vi "main.vi"() -> ()   [LabVIEW 2019]
uses:
  <vilib>/Utility/miscctls.llb/LVPointTypeDef.ctl
  GitHub/ui-tools/Engine/Move Speed.ctl
  <vilib>/numeric/Random Number (Range) U64.vi
  <vilib>/numeric/sub_Random U32.vi
  <vilib>/Utility/file.llb/Read Delimited Spreadsheet (string).vi
  <vilib>/Utility/file.llb/Write Delimited Spreadsheet (string).vi
  <vilib>/Utility/file.llb/Write Delimited Spreadsheet (I64).vi
  <vilib>/Utility/file.llb/Read Delimited Spreadsheet (I64).vi
panel:
  out "倒计时":i32(slide) scale=-1.0..2181.0
  out "x-y":i32
  in  "数组":u64[](array[numeric])
  in  "Toolbar 5":T1
  in  "WindowsMediaPlayer":refnum<k7>(container)
  in  "错误输入（无错误）":errorcluster
  in  "AniGIF":refnum<k7>(container)
  in  "键盘启用":bool
  out "游戏界面_时间到":bool
  in  "亮灯次数":i32=1
  in  "是否开始计时？":bool
  out "难度":string="困难"
  out "闪烁间隔":i32=727
  out "超时时间":i32=500
  in  "选项卡控件":T2(tab)
  in  "密码:":string
  in  "账号:":string
  in  "登录界面_修改密码":bool
  in  "登陆界面_注册":bool
  in  "登录界面_登录":bool
  in  "登录界面_退出":bool
  in  "主界面_返回":bool
  in  "主界面_进入游戏":bool
  in  "用户注册_注册":bool
  in  "用户注册_返回":bool
  in  "注册簇":T3
  in  "修改密码_返回":bool
  in  "修改密码_修改":bool
  in  "修改密码簇 2":T4
  in  "TOP10_返回":bool
  out "玩家                      积分          简单":string[][](array[string])
  out "玩家                      积分          中等":string[][](array[string])
  out "玩家                      积分          困难":string[][](array[string])
  in  "TOP10_退出":bool
  in  "游戏规则_返回":bool
  out "分数":i32
  out "游戏界面_下":T5
  out "游戏界面_右":T6
  out "游戏界面_左":T7
  out "游戏界面_上":T8
  out "难度：分数":string
  in  "游戏界面_结束":bool
  out "玩家":string
  # "游戏开始时，第一次亮一\n个灯，然后我们需要点击一次已 \n，第二次会亮两个灯，包括第一\n次的灯，第三次亮三个，每次增\n加一个灯，你都需要按顺序点击\n，或者使用键盘的↑↓←→操作"
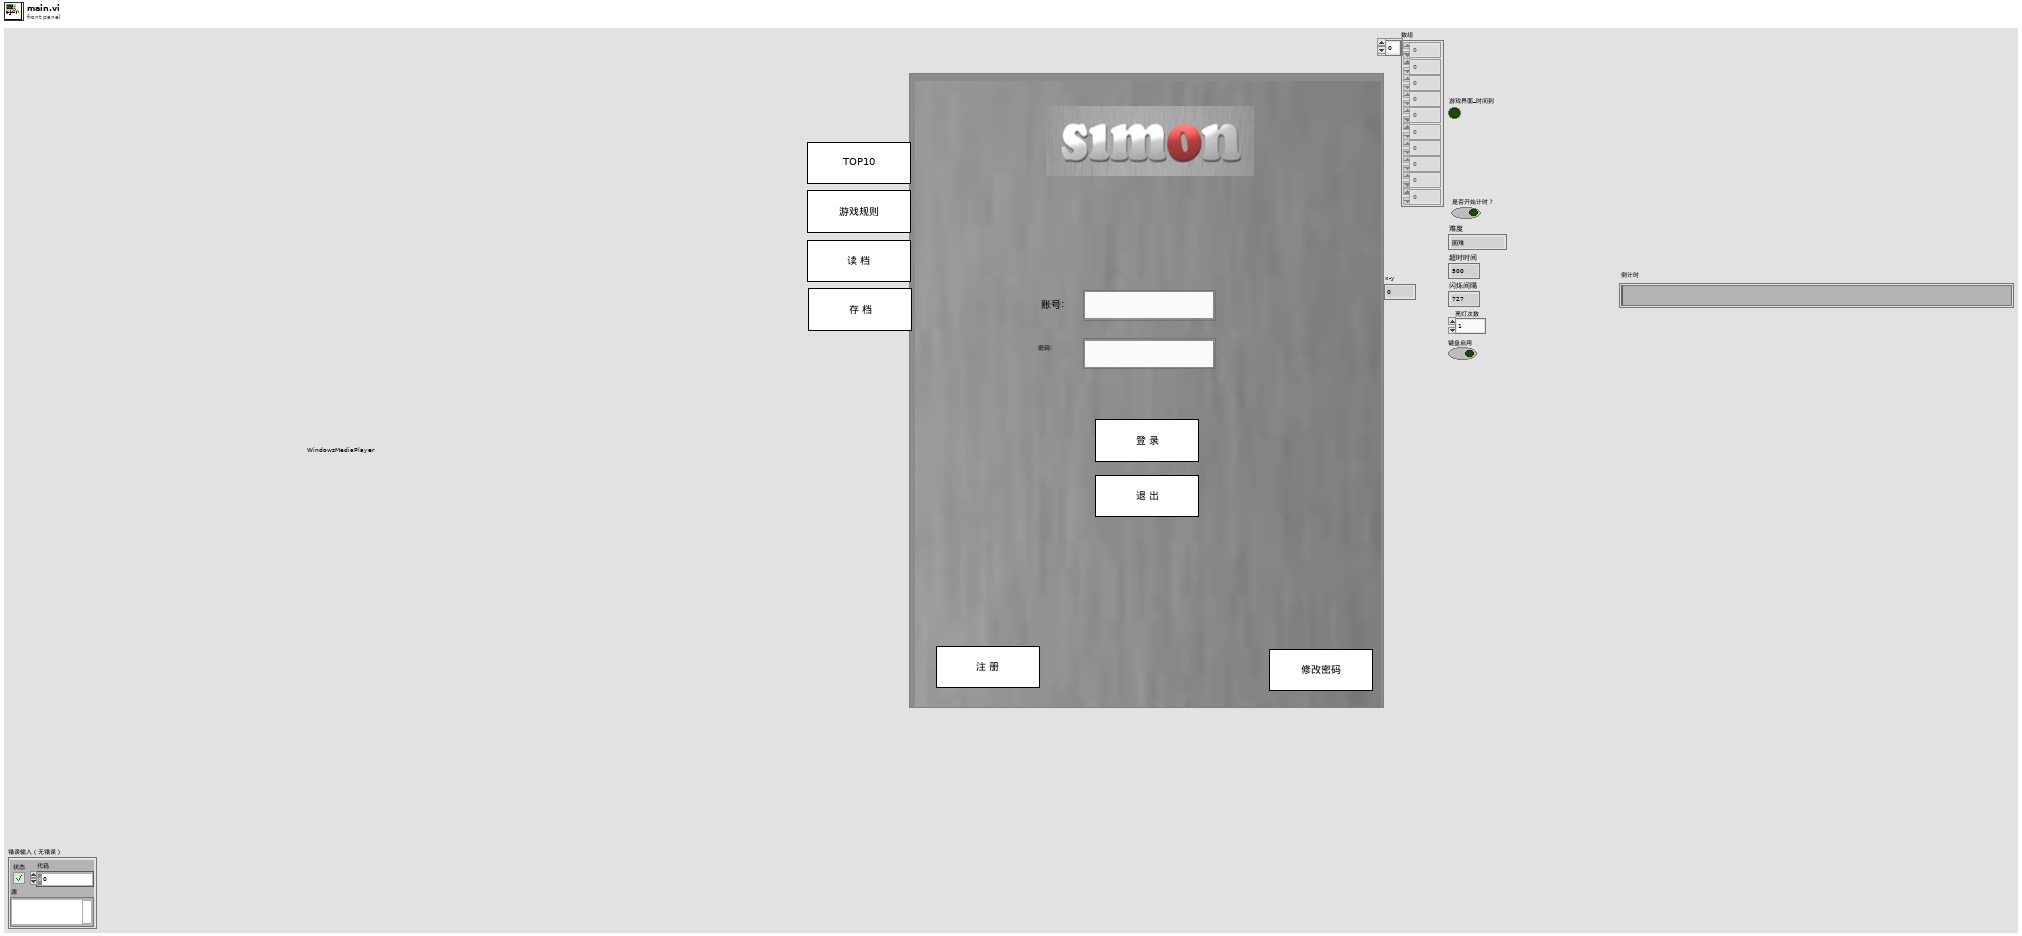
[diagram p1: front panel]
types:
  T1 = cluster{"主界面_TOP10":bool, "主界面_游戏规则":bool, "游戏界面_读档":bool, "游戏界面_存档":bool}
  T2 = enum32{"登录界面", "主界面", "用户注册", "修改密码", "TOP10", "游戏规则", "游戏界面"}
  T3 = cluster{"注册账户:":string, "注册密码:":string, "确认密码:":string}
  T4 = cluster{"账号:":string, "旧密码:":string, "新密码:":string, "确认密码:":string}
  T5 = typedef "红灯.ctl" = bool
  T6 = typedef "蓝灯.ctl" = bool
  T7 = typedef "黄灯.ctl" = bool
  T8 = typedef "绿灯.ctl" = bool
  T9 = typedef "LVPointTypeDef.ctl" = cluster{"Horizontal":i16, "Vertical":i16}
  T10 = typedef "按键枚举.ctl" = enum16{"读档", "存档", "按错", "退出", "黄", "红", "蓝", "绿"}
  T11 = typedef "选项卡枚举.ctl" = enum32{"登录界面", "主界面", "用户注册", "修改密码", "TOP10", "游戏规则", "游戏界面"}
  T12 = typedef "Move Speed.ctl" = enum16{"Normal", "Fast", "Slow", "Instantaneous"}
  T13 = enum32{"Invalid", "Standard", "Closed", "Hidden", "Minimized", "Maximized"}
  T14 = enum32{"invalid app kind", "Development System", "Run Time System", "Student Edition", "Embedded LabVIEW", "Evaluation", "Custom"}
  T15 = cluster{"Core":cluster{"Current VI Reference":refnum<vi>, "Close Panel on Exit?":bool}, "Your Boolean data":bool, "注册账户":string, "注册密码":string, "修改密码_新密码":string, "修改密码_账户":string, "用户名":string, "难度_保存":string, "亮灯次数_保存":i32, "超时时间_保存":i32, "闪烁间隔_保存":i32, "积分_保存":i32, "积分_排名":i32}
  T16 = typedef "LVRectTypeDef.ctl" = cluster{"Left":i16, "Top":i16, "Right":i16, "Bottom":i16}
  T17 = cluster{"left":i16, "top":i16, "right":i16, "bottom":i16}
  T18 = cluster{"left":i16, "top":i16, "right":i16, "bottom":i16}[]
  T19 = typedef "LVBoundsTypeDef.ctl" = cluster{"Width":u32, "Height":u32}
  T20 = typedef "eventvkey.ctl" = enum16{"ASCII", "Enter", "Return", "Shift", "Ctrl", "Alt", "Cmd", "Opt", "Caps", "NumLock", "Clear", "Break", "Up", "Down", "Left", "Right", "Insert", "Delete", "Home", "End", "PageUp", "PageDown", "Escape", "Help", "Pause", "ScrollLock", "F1", "F2", "F3", "F4", "F5", "F6", "F7", "F8", "F9", "F10", "F11", "F12", "F13", "F14", "F15", "F16", "F17", "F18", "F19", "F20", "F21", "F22", "F23", "F24", "Play", "VolumeUp", "VolumeDown", "Mute", "Two Byte Char"}
  T21 = cluster{"Current VI Reference":refnum<vi>, "Close Panel on Exit?":bool}
  T22 = enum16{"Left Button", "Center Button", "Right Button", "Window Close"}
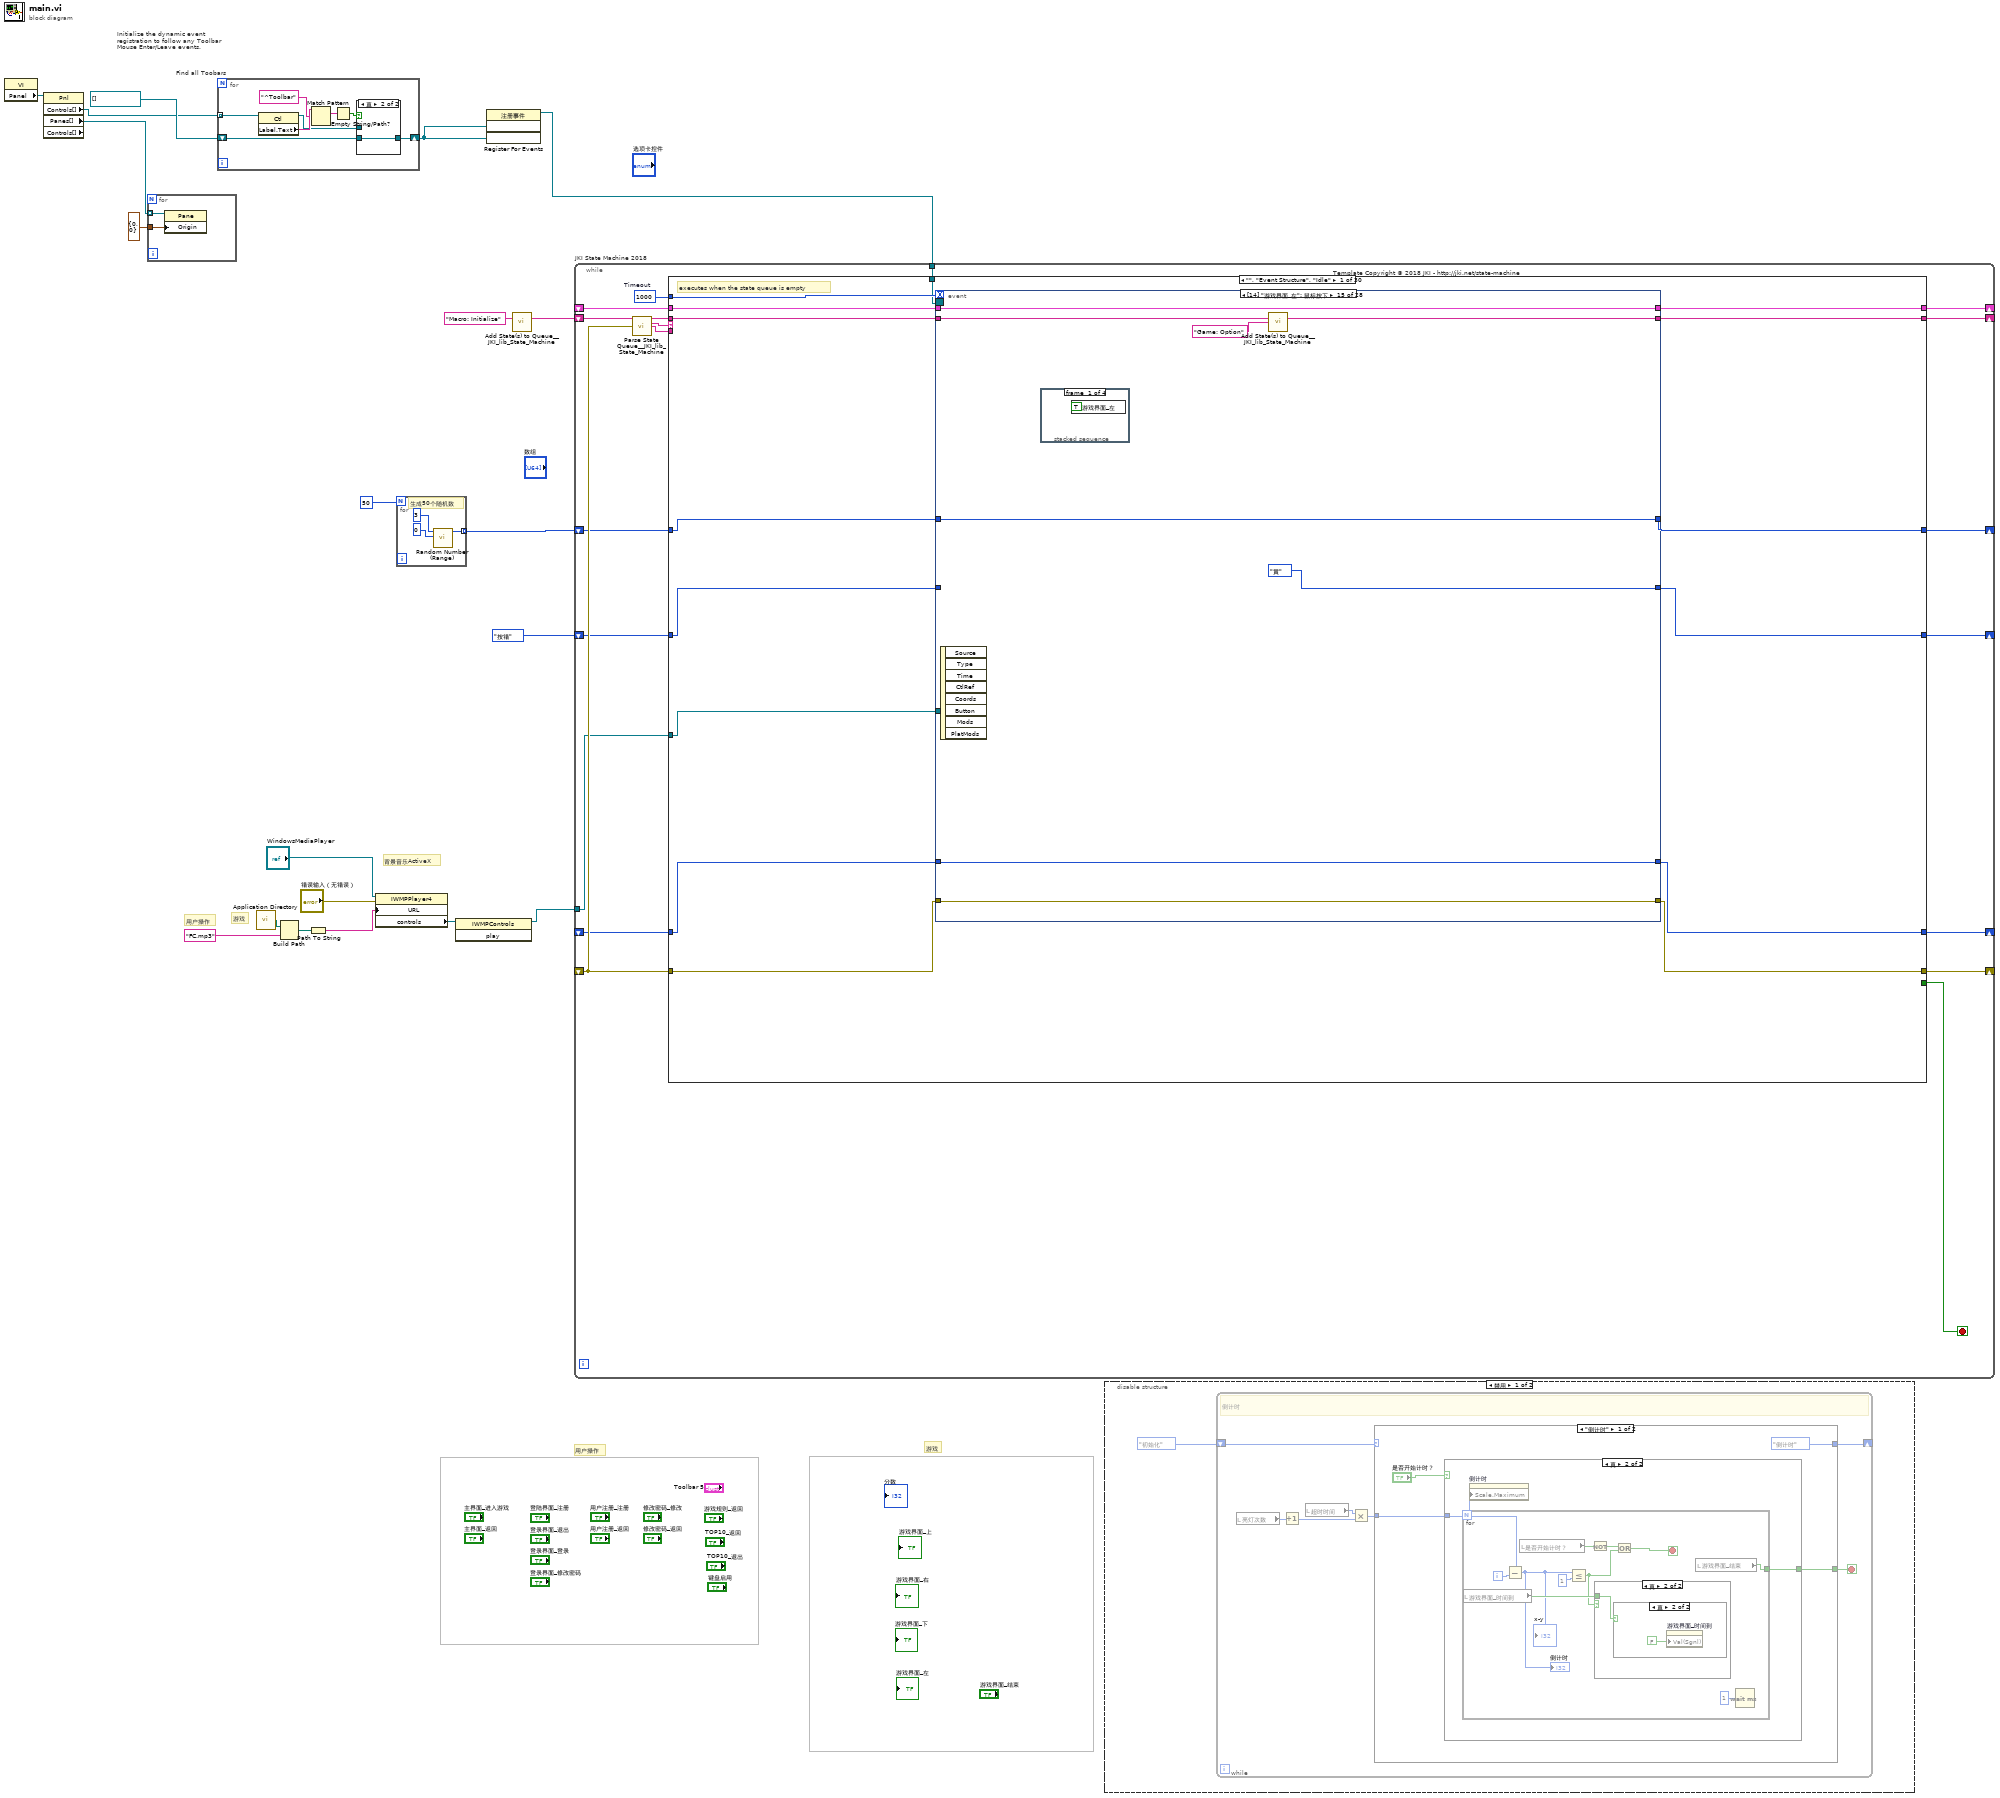
[diagram p0: block diagram]
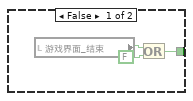
[diagram p2: hidden frame]
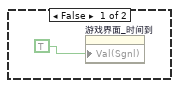
[diagram p4: hidden frame]
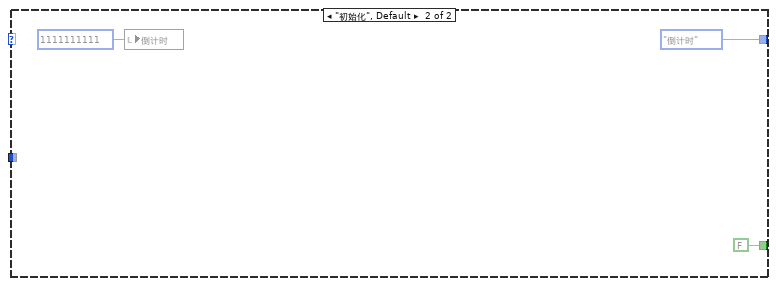
[diagram p5: hidden frame]
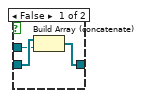
[diagram p7: hidden frame]
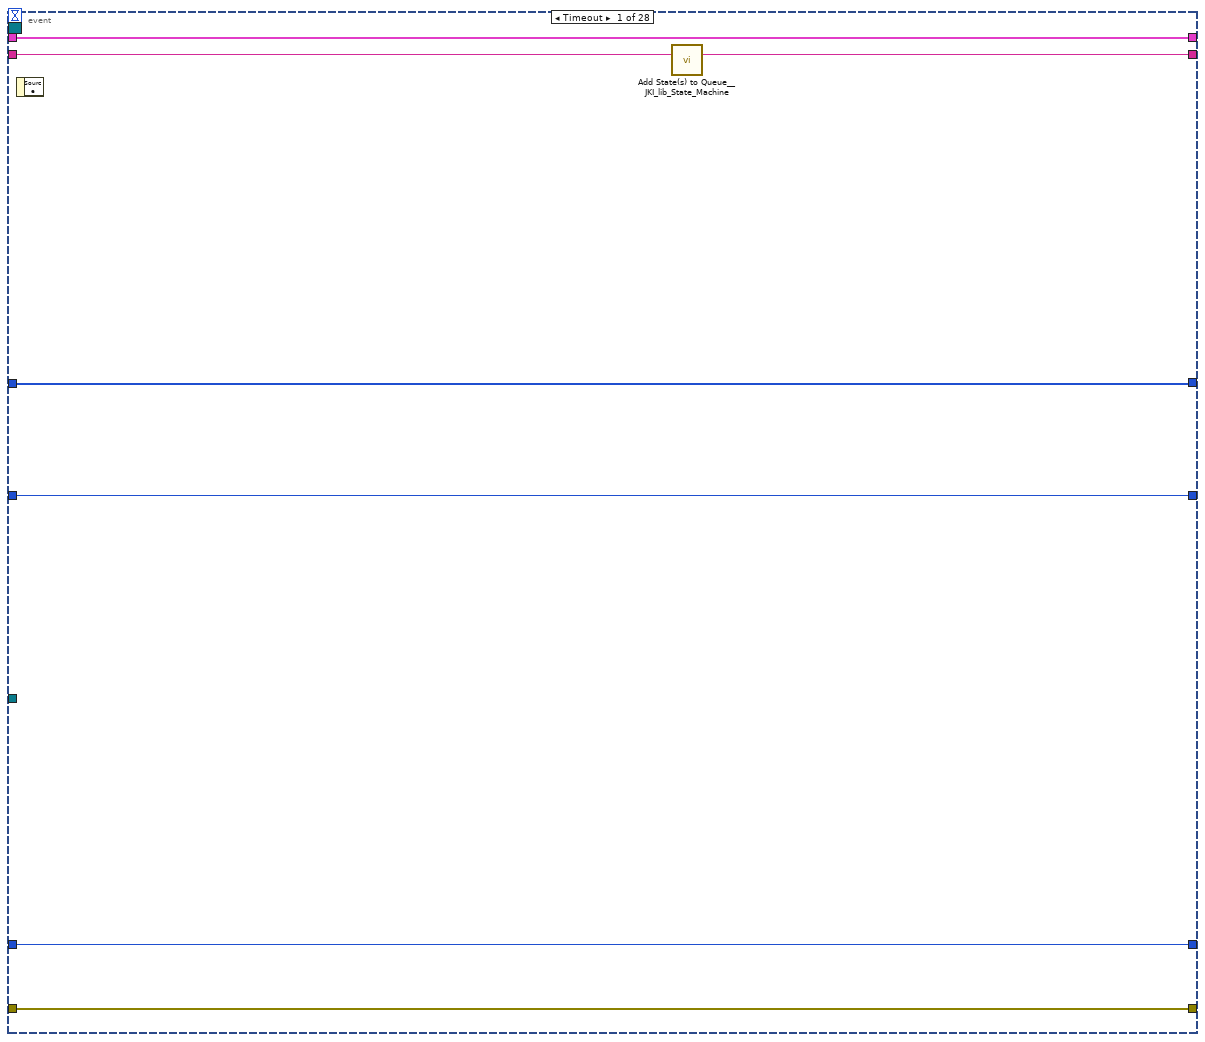
[diagram p8: hidden frame]
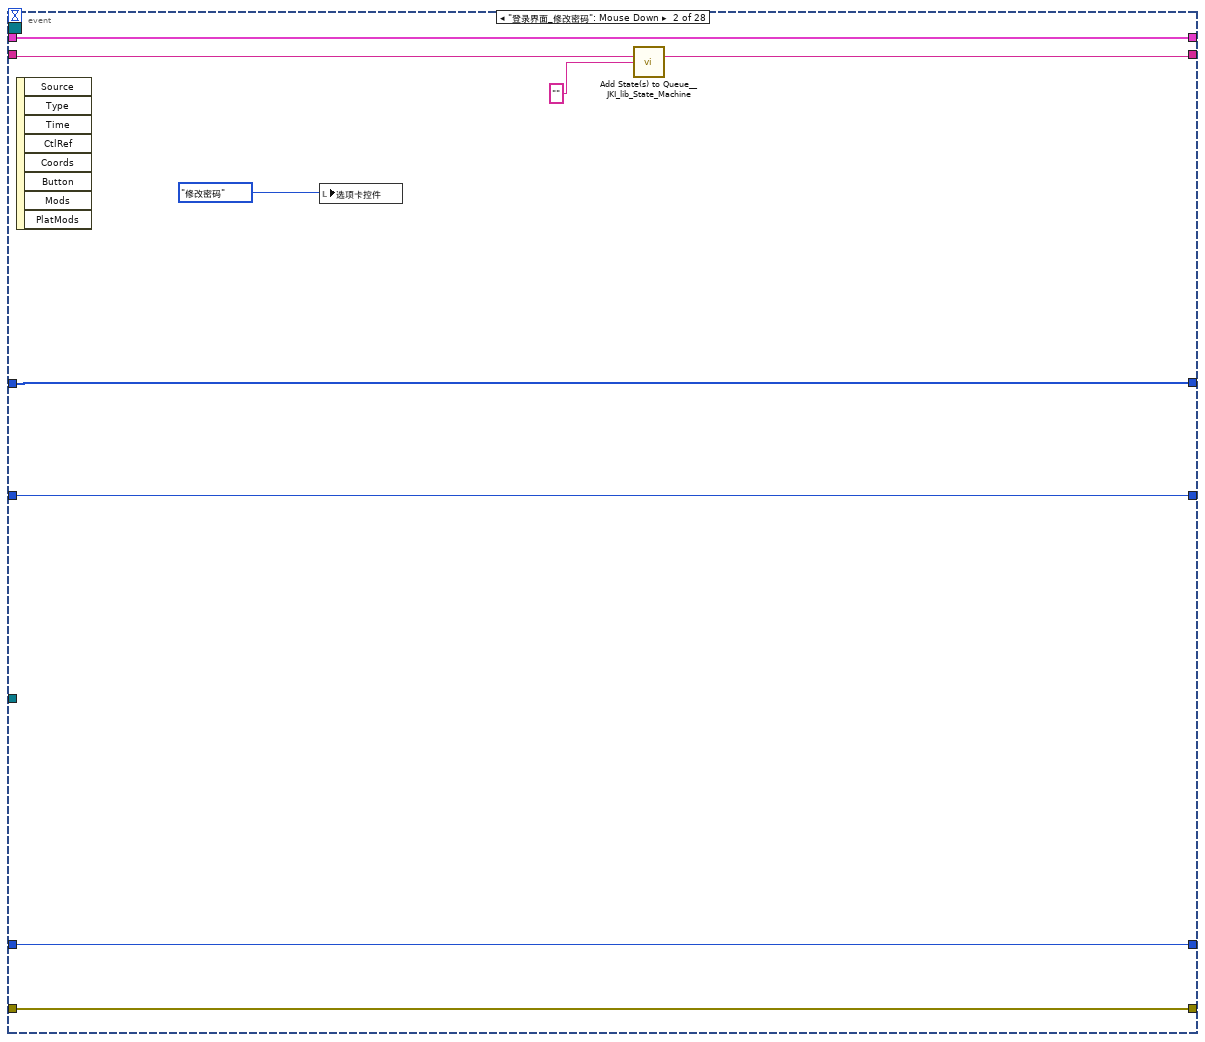
[diagram p9: hidden frame]
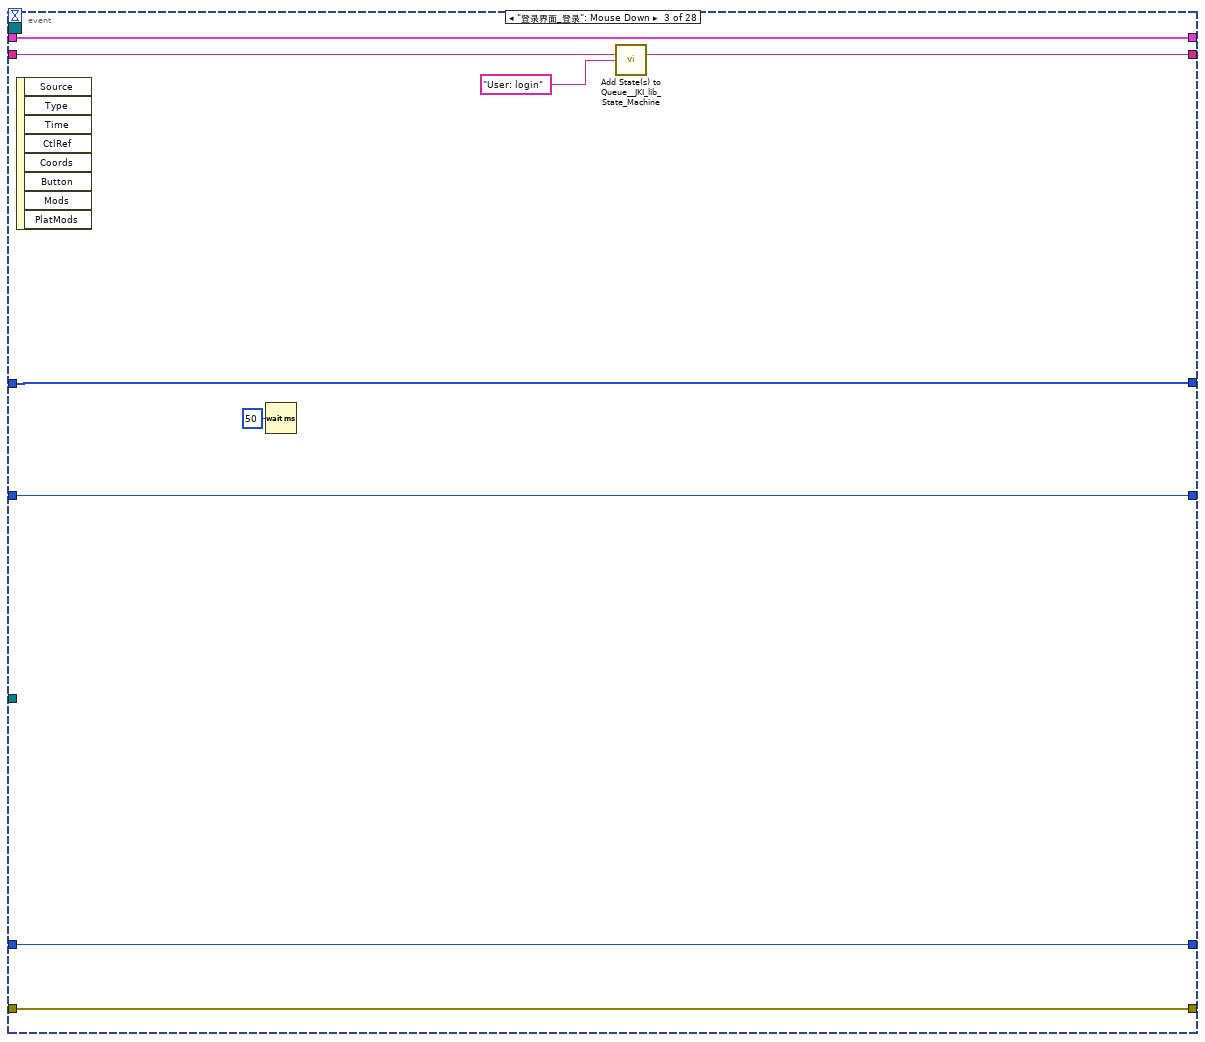
[diagram p10: hidden frame]
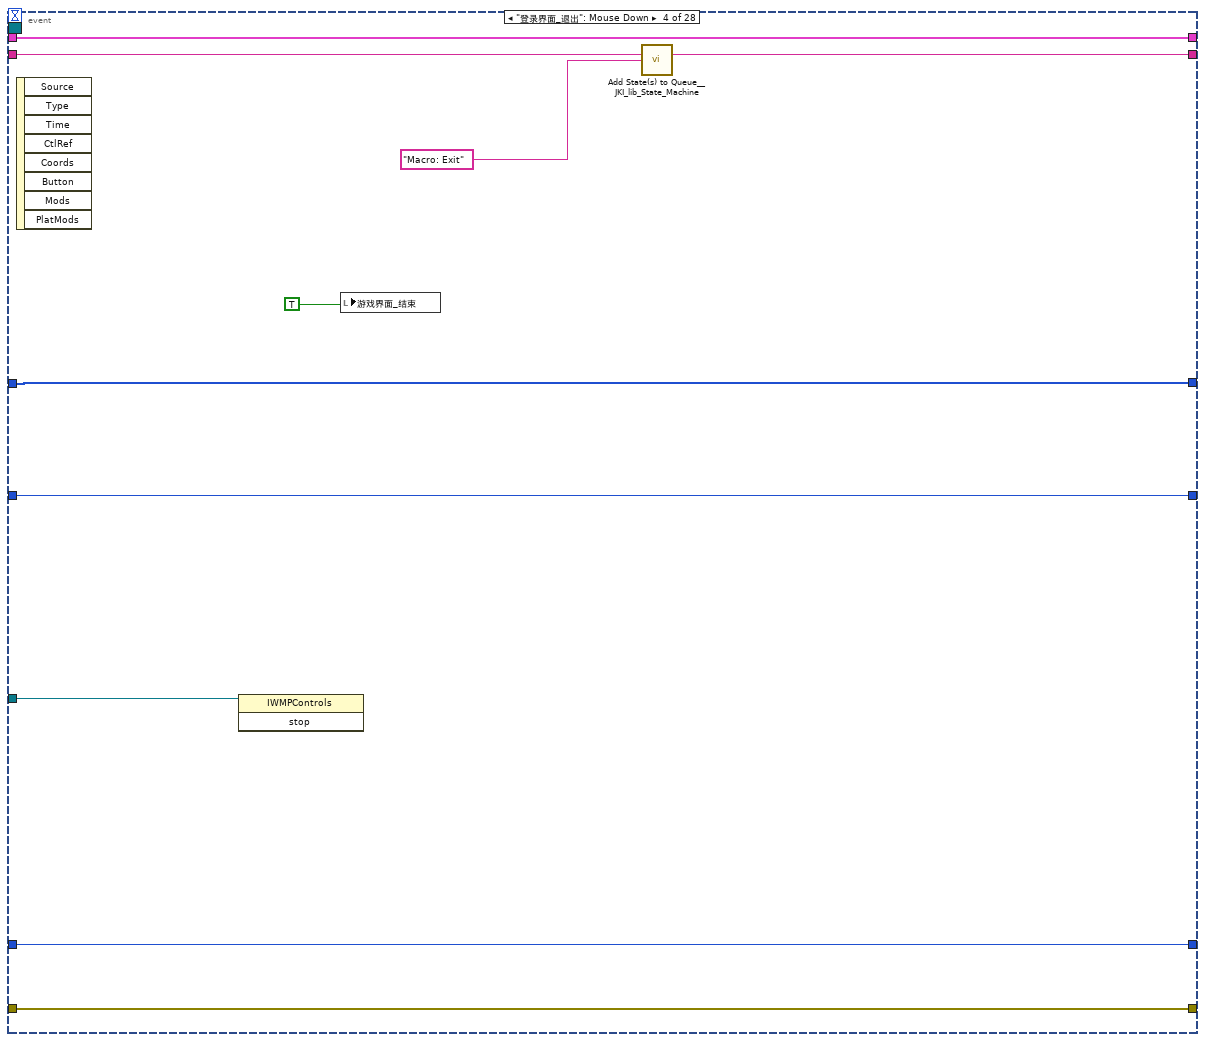
[diagram p11: hidden frame]
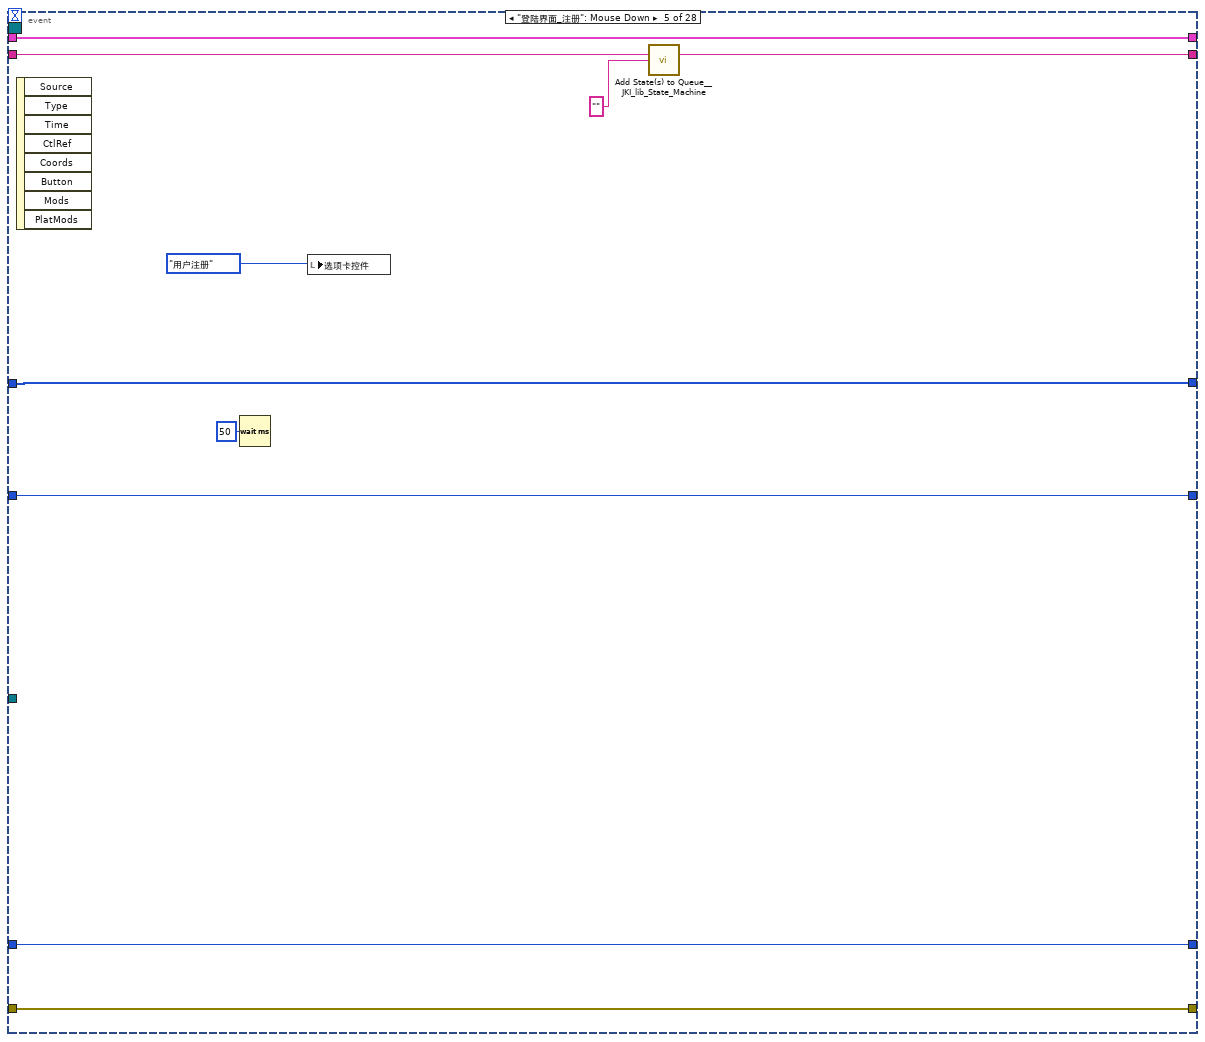
[diagram p12: hidden frame]
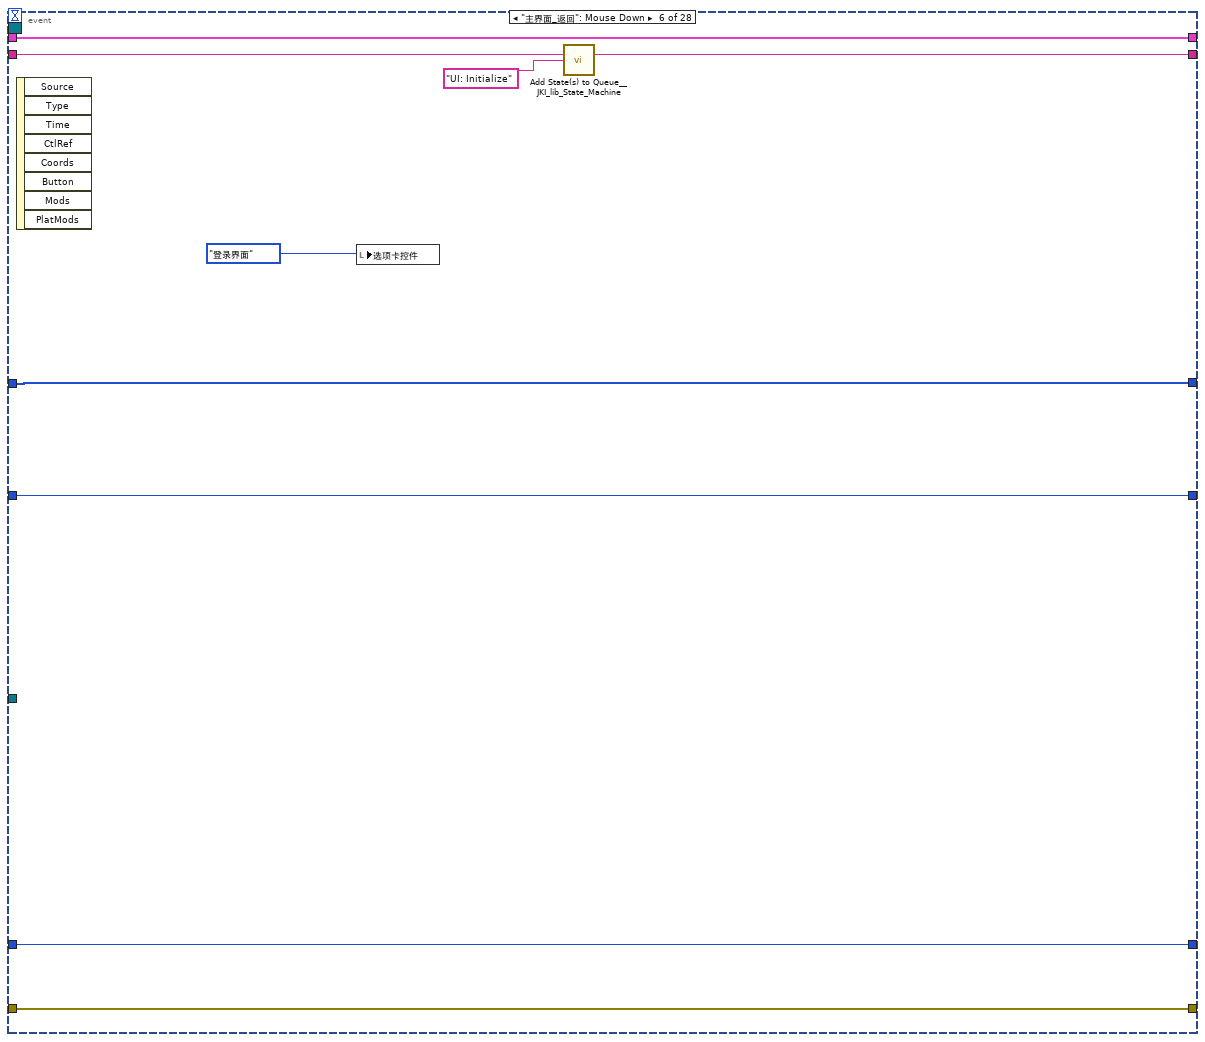
[diagram p13: hidden frame]
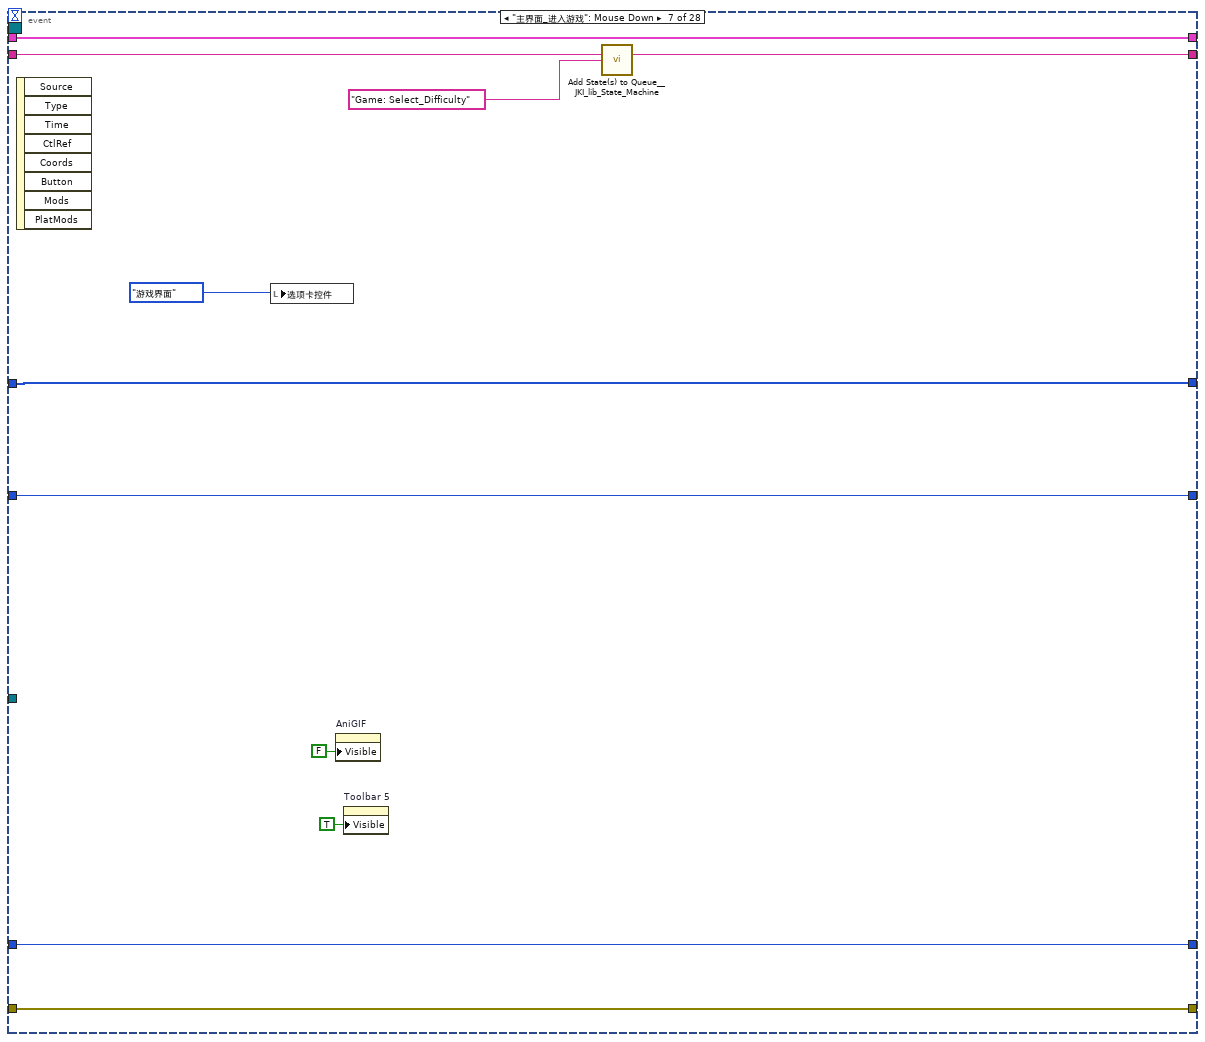
[diagram p14: hidden frame]
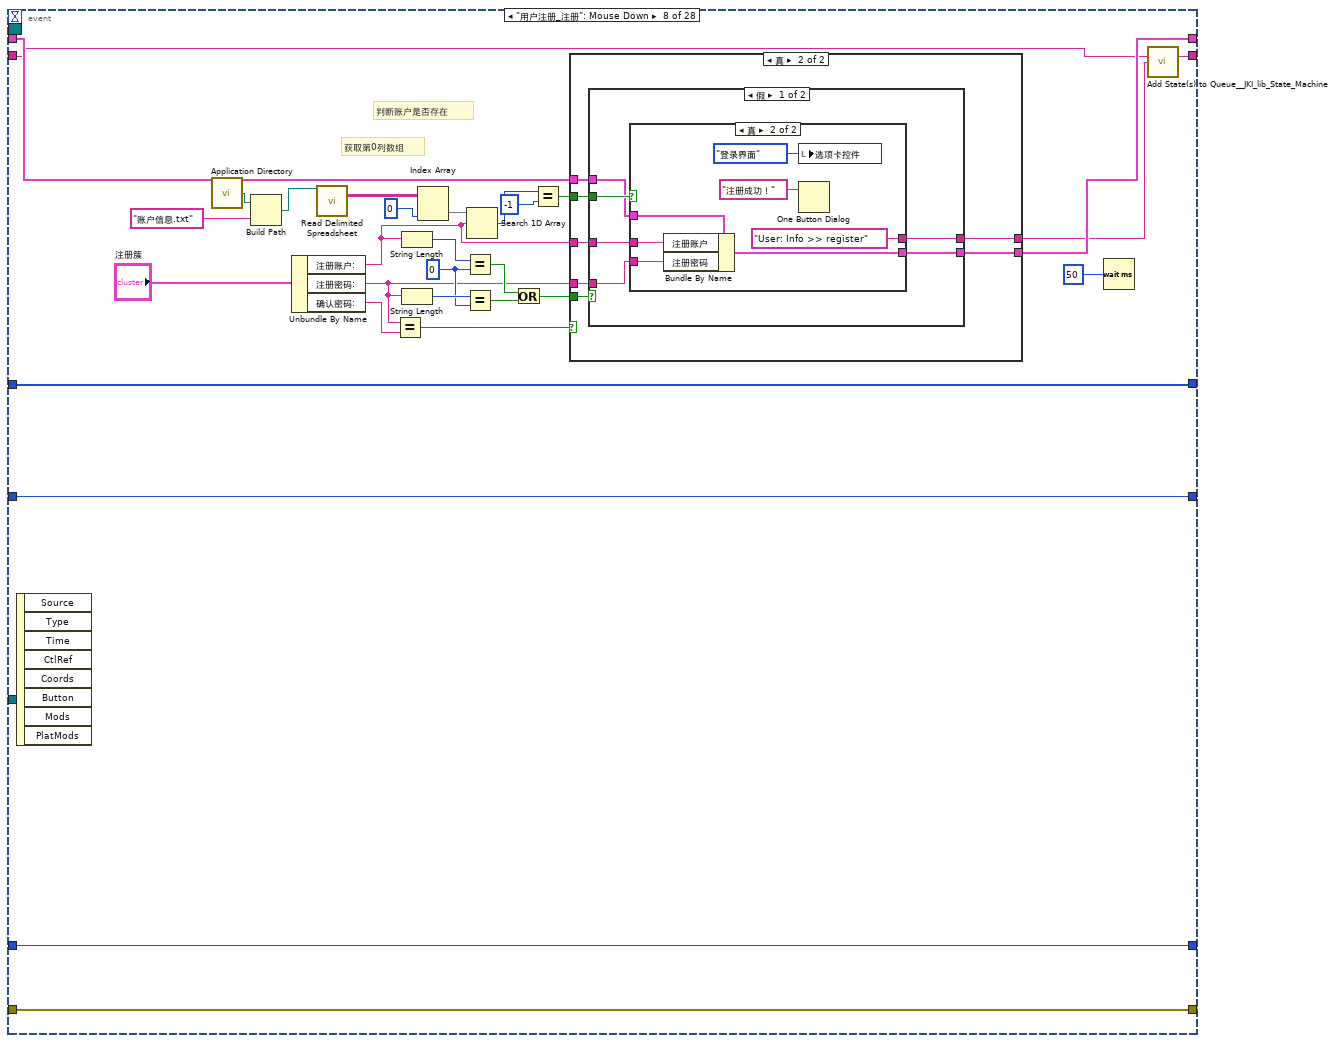
[diagram p15: hidden frame]
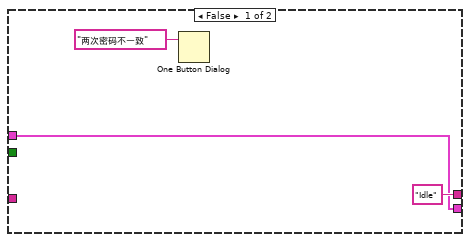
[diagram p16: hidden frame]
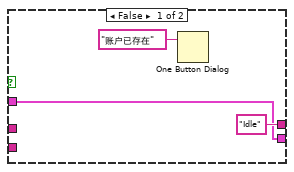
[diagram p17: hidden frame]
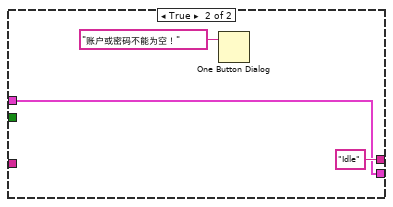
[diagram p18: hidden frame]
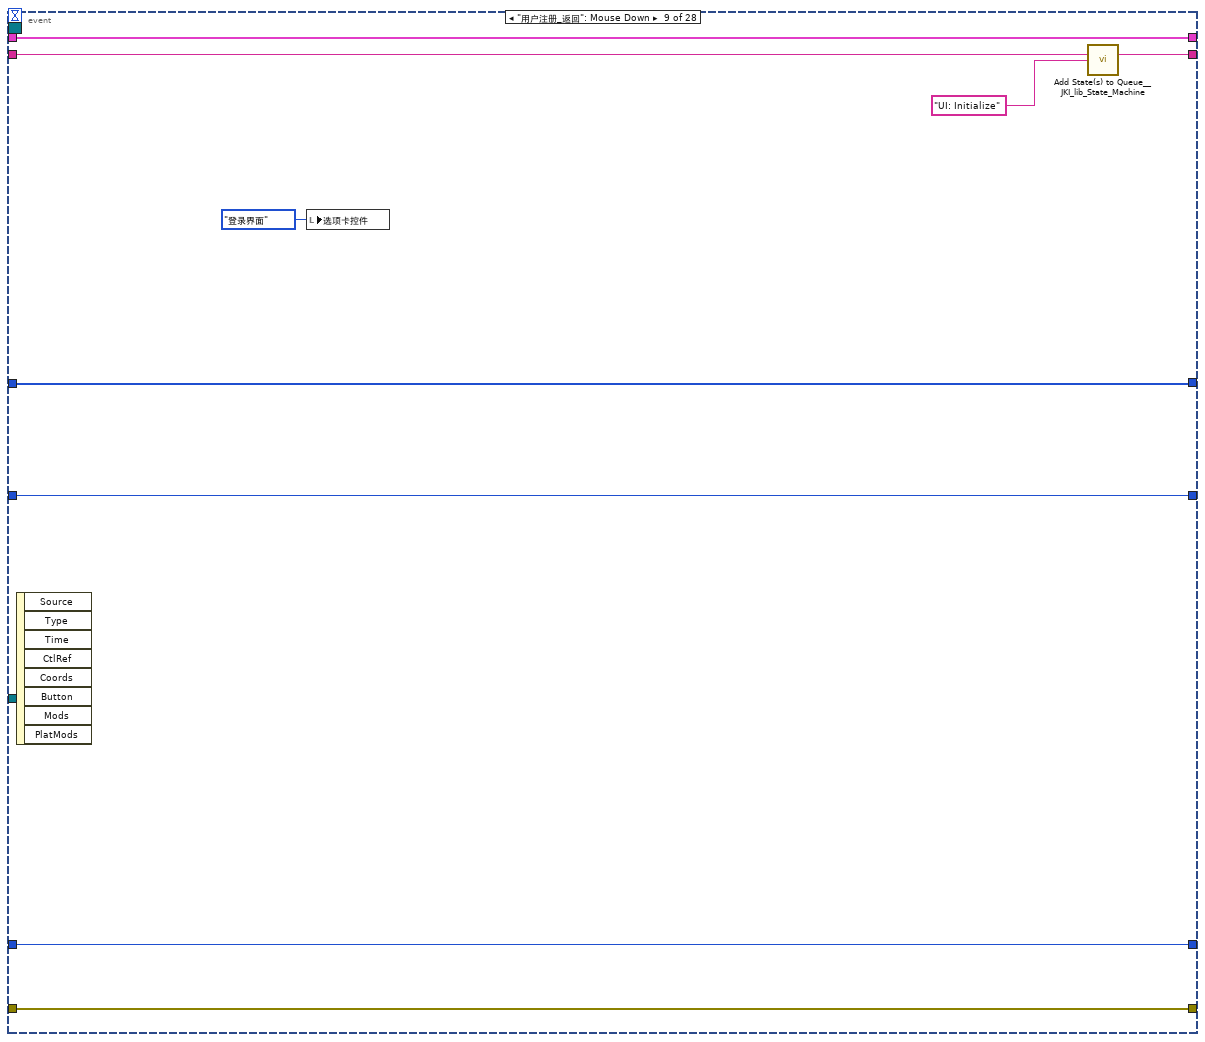
[diagram p19: hidden frame]
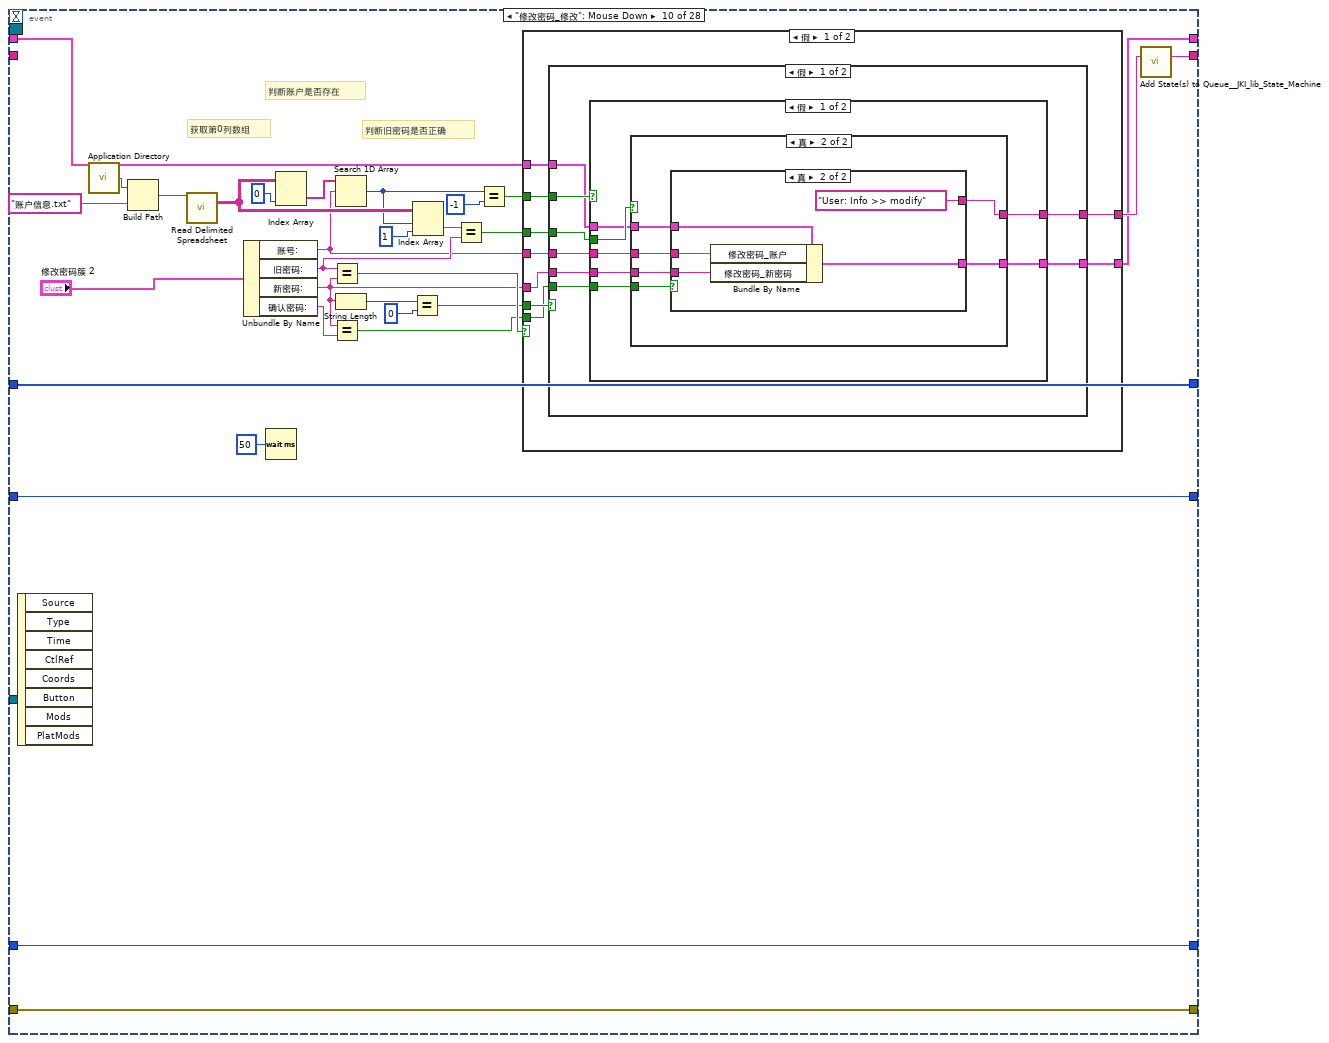
[diagram p20: hidden frame]
diagram:
  # "Find all Toobars"
  # "Initialize the dynamic event\nregistration to follow any Toolbar\nMouse Enter/Leave events."
  # "背景音乐ActiveX"
  # "游戏"
  # "用户操作"
  # "游戏"
  # "用户操作"
  n1 = property class="VI"() -> ("Panel"=w4:refnum<vi>)  [unwired: 2 in, 2 out]
  n2 = property class="Pnl" props=["Controls[]", "Panes[]", "Controls[]"](reference=w4) -> ("Controls[]"=w5:refnum<vi>[], "Panes[]"=w9:refnum<vi>[])  [unwired: 1 in, 3 out]
  n3 = for {
    tunnel: w9 -> [w21] mode=indexing
    tunnel: T9 {"Horizontal"=0, "Vertical"=0} ("Origin") -> [w22]
    n4 = property class="Pane"(reference=w21, "Origin"=w22) -> ()  [unwired: 1 in, 2 out]
  }
  n5 = for {
    tunnel: w5 -> [w23] mode=indexing
    shift-right: [w25] -> w6
    shift-left: refnum<vi>[] [] -> [w26]
    n6 = property class="Ctl"(reference=w23) -> (reference out=w24:refnum<vi>, "Label.Text"=w30:string)  [unwired: 1 in, 1 out]
    n7 = Match Pattern(string=w30, regular expression="^Toolbar") -> (match substring=w28:string)  [unwired: 4 out]
    n8 = Empty String/Path?(string/path=w28) -> (empty?=w27:bool)
    n9 = case shown="真" w27 {
      tunnel: [w31 w34] -> w25
      tunnel: w26 -> [w33 w34]
      tunnel: w24 -> [w32 _]
      frame False {
        n10 = Build Array (concatenate)(w33, w32) -> (w31:refnum<vi>[])
      }
      frame True {
      }
    }
  }
  n11 = call <vilib>:"Application Directory.vi"() -> ("Application Directory"=w11:path)
  n12 = Build Path(base path=w11, name or relative path="FC.mp3" ("名称或相对路径")) -> (appended path=w16:path)
  n13 = Path To String(path=w16) -> (string=w15:string)
  n14 = property class="IWMPPlayer4"(reference="WindowsMediaPlayer", error in="错误输入（无错误）", "URL"=w15) -> ("controls"=w13:refnum<k7>)  [unwired: 2 out]
  n15 = for {
    N: 50 -> [_]
    tunnel: [w35] -> w1 mode=indexing
    # "生成50个随机数"
    n16 = call-poly <vilib>:"Random Number (Range).vi"("lower bound (0)"=u64 0, "upper bound (100)"=u64 3) -> ("number"=w35:u64)  [unwired: 9 in]
  }
  n17 = invoke class="IWMPControls" method="play"(reference=w13) -> (reference out=w10:refnum<k7>)  [unwired: 2 in, 2 out]
  n18 = register-events(w6, w6) -> (reference out=w3:refnum<event-registration>)  [unwired: 2 in, 1 out]
  n19 = call <vilib>:"Add State(s) to Queue__JKI_lib_State_Machine.vi"("State(s) in (\"\")"="Macro: Initialize") -> ("States Out"=w20:string)  [unwired: 14 in]
  n20 = while "JKI State Machine 2018" {
    shift-right: [w49] -> _
    shift-left: _ -> [w48]
    shift-right: [w52] -> _
    shift-left: _ -> [w46]
    shift-right: [w51] -> _
    shift-left: w20 -> [w53]
    shift-right: [w44] -> _
    shift-left: w1 -> [w45]
    shift-right: [w43] -> _
    shift-left: _ -> [w42]
    shift-right: [w40] -> _
    shift-left: 按键枚举."按错" -> [w41]
    tunnel: w10 -> [w39]
    tunnel: w3 -> [w38]
    stop <- w50 stop-if-true
    w47 = 1000  # Timeout
    # "Template Copyright © 2018 JKI - http://jki.net/state-machine"
    n21 = call <vilib>:"Parse State Queue__JKI_lib_State_Machine.vi"("State Queue"=w53, "Error In (no error)"=w46) -> ("Remaining States"=w55:string, "Current State"=w56:string, "Arguments"=w54:string)  [unwired: 11 in]
    n22 = case shown="\"\", \"Event Structure\", \"Idle\"" w56 {
      selector: w56 -> [_ _ w627 _ _ _ _ _ _ _ _ _ _ _ _ _ _ _ _ _ _ _ _ _ _ _ _ _ _ _]
      tunnel: w55 -> [w71 w623 w631 w653 w662 w670 w677 w702 w711 w718 w739 w748 w762 w834 w842 w855 w862 w872 w928 w963 w970 w991 w1011 w1040 w1056 w1131 w1156 w1166 w1209 w1221]
      tunnel: w54 -> [_ _ _ _ _ _ _ _ _ _ _ w743 w756 _ _ _ _ w866 _ _ _ _ _ _ _ _ _ _ _ _]
      tunnel: w48 -> [w69 w620 w629 w646 w659 w668 w674 _ w706 w715 w737 w746 w758 w831 w839 w852 w859 w869 w906 w960 w967 w979 w1008 w1037 w1053 w1128 w1145 w1163 w1206 w1215]
      tunnel: [w68 w621 w633 w650 errorcluster {"status"=FALSE, "code"=0, "source"=""} ("error out") w667 w675 w699 w707 w716 w736 w744 w759 w832 w840 w853 w860 w870 w926 w961 w968 w989 w1009 w1038 w1054 w1129 w1154 w1164 w1207 w1219] -> w52
      tunnel: w46 -> [w67 w621 w632 w650 w658 w667 w675 w699 w708 w716 w736 w745 w760 w832 w840 w853 w860 w870 w926 w961 w968 w989 w1009 w1038 w1054 w1129 w1154 w1164 w1207 w1219]
      tunnel: [w70 w622 w630 w652 w661 w669 w676 w701 w710 w717 w738 w747 w761 w833 w841 w854 w861 w871 w927 w962 w969 w990 w1010 w1039 w1055 w1130 w1155 w1165 w1208 w1220] -> w51
      tunnel: [_ _ _ _ _ TRUE _ _ _ _ _ _ _ _ _ _ _ _ _ _ _ _ _ _ _ _ _ _ _ _] -> w50
      tunnel: [w66 w620 w629 w651 w659 w668 w674 w700 w706 w715 w737 w746 w758 w831 w839 w852 w859 w869 w905 w960 w967 w978 w1008 w1037 w1053 w1128 w1142 w1163 w1206 w1215] -> w49
      tunnel: w47 -> [w65 _ _ _ _ _ _ _ _ _ _ _ _ _ _ _ _ _ _ _ _ _ _ _ _ _ _ _ _ _]
      tunnel: w45 -> [w64 w619 w626 w640 w655 w665 w673 w686 w705 w714 w735 w742 w755 w830 w837 w845 w858 w865 w903 w959 w966 w973 w1006 w1036 w1051 w1119 w1139 w1158 _ w1218]
      tunnel: [w63 w619 w626 w640 w655 w665 w673 w686 w705 w714 w735 w742 w755 w830 w837 w845 w858 w865 w903 w959 w966 w973 w1006 w1036 w1051 w1119 w1139 w1158 w1200 w1218] -> w44
      tunnel: [w61 w618 w625 w639 w656 w664 w672 0 w704 w713 w734 w741 w754 w829 w836 w844 w857 w864 w904 w958 w965 w972 w1003 1 w1047 w1118 w1140 w1161 w1205 w1217] -> w43
      tunnel: w42 -> [w62 w618 w625 w639 w656 w664 w672 _ w704 w713 w734 w741 w754 w829 w836 w844 w857 w864 w904 w958 w965 w972 w1003 _ w1042 w1118 w1140 w1161 w1205 w1217]
      tunnel: w41 -> [w60 w617 w624 w638 w654 w663 w671 w684 w703 w712 w733 w740 w753 w828 w835 w843 w856 w863 w900 w957 w964 w971 w1001 w1032 w1041 w1112 w1138 w1160 w1204 w1216]
      tunnel: [w59 w617 w624 w638 w654 w663 w671 w684 w703 w712 w733 w740 w753 w828 w835 w843 w856 w863 w900 w957 w964 w971 w1001 w1032 w1041 w1112 w1138 w1160 w1204 w1216] -> w40
      tunnel: w39 -> [w58 _ _ _ _ _ _ _ _ _ _ _ _ _ _ _ _ _ _ _ _ _ _ _ _ _ _ _ _ _]
      tunnel: w38 -> [w57 _ _ _ _ _ _ _ _ _ _ _ _ _ _ _ _ _ _ _ _ _ _ _ _ _ _ _ _ _]
      frame "", "Event Structure", "Idle" {
        # "executes when the state queue is empty"
        n23 = event shown="[14] \"游戏界面_左\": 鼠标按下" {
          selector: w57 -> [_ _ _ _ _ _ _ _ _ _ _ _ _ _ _ _ _ _ _ _ _ _ _ _ _ _ _ _]
          dyn-events: _ -> [_ _ _ _ _ _ _ _ _ _ _ _ _ _ _ _ _ _ _ _ _ _ _ _ _ _ _ _]
          timeout: w65 -> [_ _ _ _ _ _ _ _ _ _ _ _ _ _ _ _ _ _ _ _ _ _ _ _ _ _ _ _]
          tunnel: w71 -> [w78 w85 w94 w103 w114 w122 w134 w138 w202 _ w291 w300 w311 w323 w335 w348 w355 w366 w373 w379 w390 w409 w464 w546 w556 w596 w607 w616]
          tunnel: [w77 w86 w95 w104 w115 w123 w133 w139 w203 w207 w292 w301 w312 w324 w336 w349 w356 w365 w374 w380 w391 w408 w465 w545 w557 w597 w606 w615] -> w70
          tunnel: w69 -> [w75 w87 w96 w106 w116 w125 w136 w141 w204 w208 w293 w302 w314 w326 w338 w350 w358 w367 w375 w382 w393 w410 w466 w547 w558 w595 w604 w613]
          tunnel: [w76 w83 w92 w105 w112 w124 w135 w166 w197 w235 w287 w296 w309 w320 w331 w344 w352 w363 w376 w384 w388 w404 w459 w543 w551 w594 w605 w614] -> w68
          tunnel: w67 -> [w76 w83 w92 w105 w112 w124 w135 w166 w197 w235 w287 w296 w309 w320 w331 w344 w352 w363 w376 w384 w388 w404 w459 w543 w551 w594 w605 w614]
          tunnel: [w75 w87 w96 w106 w116 w125 w136 w140 w204 w205 w293 w302 w314 w326 w338 w350 w358 w367 w375 w382 w393 w410 w466 w547 w558 w595 w604 w613] -> w66
          tunnel: w64 -> [w74 w81 w90 w100 w109 w119 w130 w163 w200 w232 w290 w297 w310 w321 w334 w347 w354 w362 w371 w383 w387 w407 w462 w542 w553 w593 w602 w610]
          tunnel: [w74 w81 w90 w100 w109 w119 w130 w163 w200 w232 w290 w297 w310 w321 w334 w347 w354 w362 w371 w383 w387 w407 w462 w542 w553 w593 w602 w610] -> w63
          tunnel: w62 -> [w73 w80 w89 w99 w108 w118 w129 w165 w198 w234 w288 w298 w307 w319 w332 w345 w351 w361 w370 w378 w386 w405 w460 w541 w552 w592 w601 w609]
          tunnel: [w73 w80 w89 w99 w108 w118 w129 w165 w198 w234 w288 w298 w307 w319 w332 w345 w351 w361 w370 w378 w386 w405 w460 w541 w552 w592 w601 w609] -> w61
          tunnel: w60 -> [w72 w79 w88 w98 w107 w117 w128 w164 w199 w233 w289 _ _ _ _ _ _ w360 w369 _ _ w406 w461 w540 w548 w591 w600 w608]
          tunnel: [w72 w79 w88 w98 w107 w117 w128 w164 w199 w233 w289 按键枚举."绿" 按键枚举."蓝" 按键枚举."红" 按键枚举."黄" 按键枚举."退出" 按键枚举."退出" w360 w369 按键枚举."存档" 按键枚举."读档" w406 w461 w540 w554 w591 w600 w608] -> w59
          tunnel: w58 -> [_ _ _ w97 _ _ _ _ _ _ _ _ _ _ _ _ _ _ _ _ _ _ _ _ _ _ _ _]
          event Timeout {
            n24 = event-data() -> ()  [unwired: 1 in, 1 out]
            n25 = call <vilib>:"Add State(s) to Queue__JKI_lib_State_Machine.vi"("State(s) in (\"\")"=w78) -> ("States Out"=w77:string)  [unwired: 14 in]
          }
          event "登录界面_修改密码": Mouse Down {
            n26 = event-data() -> ()  [unwired: 1 in, 8 out]
            n27 = local write "选项卡控件"(选项卡枚举."修改密码" ("枚举")) -> ()
            n28 = call <vilib>:"Add State(s) to Queue__JKI_lib_State_Machine.vi"("State(s) in (\"\")"=w85, "State(s) at Back (\"\")"="" ("State(s) at Back (\"\")")) -> ("States Out"=w86:string)  [unwired: 13 in]
          }
          event "登录界面_登录": Mouse Down {
            n29 = event-data() -> ()  [unwired: 1 in, 8 out]
            n30 = Wait (ms)(milliseconds to wait=u32 50 ("等待时间（毫秒）")) -> ()  [unwired: 1 out]
            n31 = call <vilib>:"Add State(s) to Queue__JKI_lib_State_Machine.vi"("State(s) in (\"\")"=w94, "State(s) at Back (\"\")"="User: login" ("State(s) at Back (\"\")")) -> ("States Out"=w95:string)  [unwired: 13 in]
          }
          event "登录界面_退出": Mouse Down {
            n32 = event-data() -> ()  [unwired: 1 in, 8 out]
            n33 = invoke class="IWMPControls" method="stop"(reference=w97) -> ()  [unwired: 2 in, 3 out]
            n34 = local write "游戏界面_结束"(TRUE ("结束")) -> ()
            n35 = call <vilib>:"Add State(s) to Queue__JKI_lib_State_Machine.vi"("State(s) in (\"\")"=w103, "State(s) at Back (\"\")"="Macro: Exit") -> ("States Out"=w104:string)  [unwired: 13 in]
          }
          event "登陆界面_注册": Mouse Down {
            n36 = event-data() -> ()  [unwired: 1 in, 8 out]
            n37 = Wait (ms)(milliseconds to wait=u32 50 ("等待时间（毫秒）")) -> ()  [unwired: 1 out]
            n38 = local write "选项卡控件"(选项卡枚举."用户注册" ("枚举")) -> ()
            n39 = call <vilib>:"Add State(s) to Queue__JKI_lib_State_Machine.vi"("State(s) in (\"\")"=w114, "State(s) at Back (\"\")"="" ("State(s) at Back (\"\")")) -> ("States Out"=w115:string)  [unwired: 13 in]
          }
          event "主界面_返回": Mouse Down {
            n40 = event-data() -> ()  [unwired: 1 in, 8 out]
            n41 = local write "选项卡控件"(选项卡枚举."登录界面" ("枚举")) -> ()
            n42 = call <vilib>:"Add State(s) to Queue__JKI_lib_State_Machine.vi"("State(s) in (\"\")"=w122, "State(s) at Back (\"\")"="UI: Initialize") -> ("States Out"=w123:string)  [unwired: 13 in]
          }
          event "主界面_进入游戏": Mouse Down {
            n43 = event-data() -> ()  [unwired: 1 in, 8 out]
            n44 = local write "选项卡控件"(选项卡枚举."游戏界面" ("枚举")) -> ()
            n45 = property on="AniGIF" class="AXCont"("Visible"=FALSE ("可见")) -> ()  [unwired: 2 in, 2 out]
            n46 = property on="Toolbar 5" class="Clust (严格)"("Visible"=TRUE ("可见")) -> ()  [unwired: 2 in, 2 out]
            n47 = call <vilib>:"Add State(s) to Queue__JKI_lib_State_Machine.vi"("State(s) in (\"\")"=w134, "State(s) at Back (\"\")"="Game: Select_Difficulty") -> ("States Out"=w133:string)  [unwired: 13 in]
          }
          event "用户注册_注册": Mouse Down {
            w149 = 0 ("y")
            # "判断账户是否存在"
            # "获取第0列数组"
            n48 = event-data() -> ()  [unwired: 1 in, 8 out]
            n49 = call <vilib>:"Application Directory.vi"() -> ("Application Directory"=w157:path)
            n50 = Build Path(base path=w157, name or relative path="账户信息.txt" ("名称或相对路径")) -> (appended path=w158:path)
            n51 = Unbundle By Name("注册簇") -> ("注册账户:"=w145:string, "注册密码:"=w144:string, "确认密码:"=w154:string)
            n52 = call-poly <vilib>:"Read Delimited Spreadsheet.vi"("file path (dialog if empty)"=w158) -> ("all rows"=w159:string[][])  [unwired: 9 in, 5 out]
            n53 = Equal?(x=w144, y=w154) -> (x = y?=w162:bool)
            n54 = String Length(string=w145) -> (length=w150:i32)
            n55 = String Length(string=w144) -> (length=w161:i32)
            n56 = Index Array(array=w159, index (col)=0 ("禁用的索引 (列)")) -> (element=w160:string[])  [unwired: 1 in]
            n57 = Equal?(x=w150, y=w149) -> (x = y?=w147:bool)
            n58 = Equal?(x=w161, y=w149) -> (x = y?=w148:bool)
            n59 = Search 1D Array(1D array=w160, element=w145) -> (index of element=w153:i32)  [unwired: 1 in]
            n60 = Or(x=w147, y=w148) -> (x .or. y?=w146:bool)
            n61 = Equal?(x=w153, y=-1) -> (x = y?=w151:bool)
            n62 = case shown="真" w162 {
              tunnel: ["Idle" w175] -> w137
              tunnel: w146 -> [_ w176]
              tunnel: w151 -> [_ w174]
              tunnel: w141 -> [w167 w173]
              tunnel: w145 -> [_ w172]
              tunnel: w144 -> [_ w171]
              tunnel: [w167 w170] -> w140
              frame False {
                n63 = One Button Dialog(message="两次密码不一致" ("消息")) -> ()  [unwired: 1 in, 1 out]
              }
              frame True {
                n64 = case shown="假" w176 {
                  tunnel: [w181 "Idle"] -> w175
                  tunnel: w174 -> [w182 _]
                  tunnel: w173 -> [w180 w193]
                  tunnel: w172 -> [w179 _]
                  tunnel: w171 -> [w178 _]
                  tunnel: [w177 w193] -> w170
                  frame False {
                    n65 = case shown="真" w182 {
                      tunnel: ["Idle" "User: Info >> register"] -> w181
                      tunnel: w180 -> [w183 w190]
                      tunnel: w179 -> [_ w189]
                      tunnel: w178 -> [_ w188]
                      tunnel: [w183 w187] -> w177
                      frame False {
                        n66 = One Button Dialog(message="账户已存在" ("消息")) -> ()  [unwired: 1 in, 1 out]
                      }
                      frame True {
                        n67 = Bundle By Name(cluster=w190, "注册账户"=w189, "注册密码"=w188) -> (w187:T15)
                        n68 = local write "选项卡控件"(选项卡枚举."登录界面" ("枚举")) -> ()
                        n69 = One Button Dialog(message="注册成功！" ("消息")) -> ()  [unwired: 1 in, 1 out]
                      }
                    }
                  }
                  frame True {
                    n70 = One Button Dialog(message="账户或密码不能为空！" ("消息")) -> ()  [unwired: 1 in, 1 out]
                  }
                }
              }
            }
            n71 = Wait (ms)(milliseconds to wait=u32 50 ("等待时间（毫秒）")) -> ()  [unwired: 1 out]
            n72 = call <vilib>:"Add State(s) to Queue__JKI_lib_State_Machine.vi"("State(s) in (\"\")"=w138, "State(s) at Back (\"\")"=w137) -> ("States Out"=w139:string)  [unwired: 13 in]
          }
          event "用户注册_返回": Mouse Down {
            n73 = event-data() -> ()  [unwired: 1 in, 8 out]
            n74 = local write "选项卡控件"(选项卡枚举."登录界面" ("枚举")) -> ()
            n75 = call <vilib>:"Add State(s) to Queue__JKI_lib_State_Machine.vi"("State(s) in (\"\")"=w202, "State(s) at Back (\"\")"="UI: Initialize" ("State(s) at Back (\"\")")) -> ("States Out"=w203:string)  [unwired: 13 in]
          }
          event "修改密码_修改": Mouse Down {
            # "判断旧密码是否正确"
            # "判断账户是否存在"
            # "获取第0列数组"
            n76 = event-data() -> ()  [unwired: 1 in, 8 out]
            n77 = call <vilib>:"Application Directory.vi"() -> ("Application Directory"=w230:path)
            n78 = Build Path(base path=w230, name or relative path="账户信息.txt" ("名称或相对路径")) -> (appended path=w229:path)
            n79 = call-poly <vilib>:"Read Delimited Spreadsheet.vi"("file path (dialog if empty)"=w229) -> ("all rows"=w224:string[][])  [unwired: 9 in, 5 out]
            n80 = Unbundle By Name("修改密码簇 2") -> ("账号:"=w212:string, "旧密码:"=w220:string, "新密码:"=w210:string, "确认密码:"=w214:string)
            n81 = Wait (ms)(milliseconds to wait=u32 50 ("等待时间（毫秒）")) -> ()  [unwired: 1 out]
            n82 = Index Array(array=w224, index (col)=0 ("禁用的索引 (列)")) -> (element=w226:string[])  [unwired: 1 in]
            n83 = Equal?(x=w220, y=w210) -> (x = y?=w227:bool)
            n84 = Equal?(x=w210, y=w214) -> (x = y?=w213:bool)
            n85 = Search 1D Array(1D array=w226, element=w212) -> (index of element=w223:i32)  [unwired: 1 in]
            n86 = String Length(string=w210) -> (length=w219:i32)
            n87 = Equal?(x=w219, y=0) -> (x = y?=w217:bool)
            n88 = Index Array(array=w224, index (row)=w223, index (col)=1 ("禁用的索引 (列)")) -> (element=w221:string)
            n89 = Equal?(x=w221, y=w220) -> (x = y?=w215:bool)
            n90 = Equal?(x=w223, y=-1) -> (x = y?=w216:bool)
            n91 = case shown="假" w227 {
              tunnel: [w243 "" ("消息")] -> w206
              tunnel: w217 -> [w244 _]
              tunnel: w216 -> [w242 _]
              tunnel: w215 -> [w241 _]
              tunnel: w208 -> [w240 w283]
              tunnel: w210 -> [w239 _]
              tunnel: [w238 w283] -> w205
              tunnel: w213 -> [w237 _]
              tunnel: w212 -> [w236 _]
              frame False {
                n92 = case shown="假" w244 {
                  tunnel: [w251 "" ("消息")] -> w243
                  tunnel: w242 -> [w252 _]
                  tunnel: w241 -> [w250 _]
                  tunnel: w240 -> [w249 w280]
                  tunnel: w239 -> [w248 _]
                  tunnel: [w247 w280] -> w238
                  tunnel: w237 -> [w246 _]
                  tunnel: w236 -> [w245 _]
                  frame False {
                    n93 = case shown="假" w252 {
                      tunnel: [w258 "" ("消息")] -> w251
                      tunnel: w250 -> [w259 _]
                      tunnel: w249 -> [w257 w277]
                      tunnel: w248 -> [w256 _]
                      tunnel: [w255 w277] -> w247
                      tunnel: w246 -> [w254 _]
                      tunnel: w245 -> [w253 _]
                      frame False {
                        n94 = case shown="真" w259 {
                          tunnel: ["" ("消息") w267] -> w258
                          tunnel: w257 -> [w260 w266]
                          tunnel: w256 -> [_ w265]
                          tunnel: [w260 w264] -> w255
                          tunnel: w254 -> [_ w268]
                          tunnel: w253 -> [_ w263]
                          frame False {
                            n95 = One Button Dialog(message="账户或密码错误" ("消息")) -> ()  [unwired: 1 in, 1 out]
                          }
                          frame True {
                            n96 = case shown="真" w268 {
                              tunnel: ["" ("消息") "User: Info >> modify" ("消息")] -> w267
                              tunnel: w266 -> [w269 w275]
                              tunnel: w265 -> [_ w274]
                              tunnel: [w269 w273] -> w264
                              tunnel: w263 -> [_ w272]
                              frame False {
                                n97 = One Button Dialog(message="两次密码不一致" ("消息")) -> ()  [unwired: 1 in, 1 out]
                              }
                              frame True {
                                n98 = Bundle By Name(cluster=w275, "修改密码_账户"=w272, "修改密码_新密码"=w274) -> (w273:T15)
                              }
                            }
                          }
                        }
                      }
                      frame True {
                        n99 = One Button Dialog(message="用户不存在" ("消息")) -> ()  [unwired: 1 in, 1 out]
                      }
                    }
                  }
                  frame True {
                    n100 = One Button Dialog(message="新密码不能为空" ("消息")) -> ()  [unwired: 1 in, 1 out]
                  }
                }
              }
              frame True {
                n101 = One Button Dialog(message="新密码与旧密码不能相同" ("消息")) -> ()  [unwired: 1 in, 1 out]
              }
            }
            n102 = call <vilib>:"Add State(s) to Queue__JKI_lib_State_Machine.vi"("State(s) in (\"\")"=w206) -> ("States Out"=w207:string)  [unwired: 14 in]
          }
          event "修改密码_返回": Mouse Down {
            n103 = event-data() -> ()  [unwired: 1 in, 8 out]
            n104 = local write "选项卡控件"(选项卡枚举."登录界面" ("枚举")) -> ()
            n105 = call <vilib>:"Add State(s) to Queue__JKI_lib_State_Machine.vi"("State(s) in (\"\")"=w291, "State(s) at Back (\"\")"="UI: Initialize" ("State(s) at Back (\"\")")) -> ("States Out"=w292:string)  [unwired: 13 in]
          }
          event Mouse Down {
            n106 = event-data() -> ()  [unwired: 1 in, 8 out]
            n107 = stacked-sequence {
              frame #0 {
                n108 = local write "游戏界面_上"(TRUE ("上")) -> ()
              }
              frame #1 {
                n109 = Wait (ms)(milliseconds to wait=u32 60 ("等待时间（毫秒）")) -> ()  [unwired: 1 out]
              }
              frame #2 {
                n110 = local write "游戏界面_上"(FALSE ("上")) -> ()
              }
              frame #3 {
                n111 = Wait (ms)(milliseconds to wait=u32 60 ("等待时间（毫秒）")) -> ()  [unwired: 1 out]
              }
            }
            n112 = call <vilib>:"Add State(s) to Queue__JKI_lib_State_Machine.vi"("State(s) in (\"\")"=w300, "State(s) at Back (\"\")"="Game: Option" ("State(s) at Back (\"\")")) -> ("States Out"=w301:string)  [unwired: 13 in]
          }
          event Mouse Down {
            n113 = event-data() -> ()  [unwired: 1 in, 8 out]
            n114 = stacked-sequence {
              frame #0 {
                n115 = local write "游戏界面_右"(TRUE ("上")) -> ()
              }
              frame #1 {
                n116 = Wait (ms)(milliseconds to wait=u32 60 ("等待时间（毫秒）")) -> ()  [unwired: 1 out]
              }
              frame #2 {
                n117 = local write "游戏界面_右"(FALSE ("上")) -> ()
              }
              frame #3 {
                n118 = Wait (ms)(milliseconds to wait=u32 60 ("等待时间（毫秒）")) -> ()  [unwired: 1 out]
              }
            }
            n119 = call <vilib>:"Add State(s) to Queue__JKI_lib_State_Machine.vi"("State(s) in (\"\")"=w311, "State(s) at Back (\"\")"="Game: Option" ("State(s) at Back (\"\")")) -> ("States Out"=w312:string)  [unwired: 13 in]
          }
          event Mouse Down {
            n120 = event-data() -> ()  [unwired: 1 in, 8 out]
            n121 = stacked-sequence {
              frame #0 {
                n122 = local write "游戏界面_下"(TRUE ("上")) -> ()
              }
              frame #1 {
                n123 = Wait (ms)(milliseconds to wait=u32 60 ("等待时间（毫秒）")) -> ()  [unwired: 1 out]
              }
              frame #2 {
                n124 = local write "游戏界面_下"(FALSE ("上")) -> ()
              }
              frame #3 {
                n125 = Wait (ms)(milliseconds to wait=u32 60 ("等待时间（毫秒）")) -> ()  [unwired: 1 out]
              }
            }
            n126 = call <vilib>:"Add State(s) to Queue__JKI_lib_State_Machine.vi"("State(s) in (\"\")"=w323, "State(s) at Back (\"\")"="Game: Option" ("State(s) at Back (\"\")")) -> ("States Out"=w324:string)  [unwired: 13 in]
          }
          event Mouse Down {
            n127 = event-data() -> ()  [unwired: 1 in, 8 out]
            n128 = stacked-sequence {
              frame #0 {
                n129 = local write "游戏界面_左"(TRUE ("上")) -> ()
              }
              frame #1 {
                n130 = Wait (ms)(milliseconds to wait=u32 60 ("等待时间（毫秒）")) -> ()  [unwired: 1 out]
              }
              frame #2 {
                n131 = local write "游戏界面_左"(FALSE ("上")) -> ()
              }
              frame #3 {
                n132 = Wait (ms)(milliseconds to wait=u32 60 ("等待时间（毫秒）")) -> ()  [unwired: 1 out]
              }
            }
            n133 = call <vilib>:"Add State(s) to Queue__JKI_lib_State_Machine.vi"("State(s) in (\"\")"=w335, "State(s) at Back (\"\")"="Game: Option" ("State(s) at Back (\"\")")) -> ("States Out"=w336:string)  [unwired: 13 in]
          }
          event "游戏界面_时间到": Value Change {
            n134 = event-data() -> ()  [unwired: 1 in, 6 out]
            n135 = call <vilib>:"Add State(s) to Queue__JKI_lib_State_Machine.vi"("State(s) in (\"\")"=w348, "State(s) at Back (\"\")"="Game: Option" ("State(s) at Back (\"\")")) -> ("States Out"=w349:string)  [unwired: 13 in]
          }
          event "游戏界面_结束": Mouse Down {
            n136 = event-data() -> ()  [unwired: 1 in, 8 out]
            n137 = call <vilib>:"Add State(s) to Queue__JKI_lib_State_Machine.vi"("State(s) in (\"\")"=w355, "State(s) at Back (\"\")"="Game: Option" ("State(s) at Back (\"\")")) -> ("States Out"=w356:string)  [unwired: 13 in]
          }
          event "Toolbar 5.主界面_游戏规则": Mouse Down {
            n138 = event-data() -> ()  [unwired: 1 in, 8 out]
            n139 = property on="AniGIF" class="AXCont"("Visible"=FALSE ("可见")) -> ()  [unwired: 2 in, 2 out]
            n140 = local write "选项卡控件"(选项卡枚举."游戏规则" ("枚举")) -> ()
            n141 = call <vilib>:"Add State(s) to Queue__JKI_lib_State_Machine.vi"("State(s) in (\"\")"=w366) -> ("States Out"=w365:string)  [unwired: 14 in]
          }
          event "Toolbar 5.主界面_TOP10": Mouse Down {
            n142 = event-data() -> ()  [unwired: 1 in, 8 out]
            n143 = local write "选项卡控件"(选项卡枚举."TOP10" ("枚举")) -> ()
            n144 = property on="AniGIF" class="AXCont"("Visible"=FALSE ("可见")) -> ()  [unwired: 2 in, 2 out]
            n145 = call <vilib>:"Add State(s) to Queue__JKI_lib_State_Machine.vi"("State(s) in (\"\")"=w373) -> ("States Out"=w374:string)  [unwired: 14 in]
          }
          event "Toolbar 5.游戏界面_存档": Mouse Down {
            n146 = event-data() -> ()  [unwired: 1 in, 8 out]
            n147 = local write "是否开始计时？"(FALSE ("是否开始计时？")) -> ()
            n148 = call <vilib>:"Add State(s) to Queue__JKI_lib_State_Machine.vi"("State(s) in (\"\")"=w379, "State(s) at Back (\"\")"="Game: Option" ("State(s) at Back (\"\")")) -> ("States Out"=w380:string)  [unwired: 13 in]
          }
          event "Toolbar 5.游戏界面_读档": Mouse Down {
            n149 = event-data() -> ()  [unwired: 1 in, 8 out]
            n150 = call <vilib>:"Add State(s) to Queue__JKI_lib_State_Machine.vi"("State(s) in (\"\")"=w390, "State(s) at Back (\"\")"="Game: Option" ("State(s) at Back (\"\")")) -> ("States Out"=w391:string)  [unwired: 13 in]
          }
          event Mouse Enter {
            # "Find Closest border"
            n151 = event-data() -> ("CtlRef"=w394:refnum<vi>)  [unwired: 1 in, 3 out]
            n152 = property class="VI"() -> ("Front Panel.PanelBounds"=w395:T16)  [unwired: 2 in, 2 out]
            n153 = call "Calculate_GObject_Rectangle.vi"("GObject ref"=w394) -> ("Rectangle"=w401:T17, "GObject ref dup"=w396:refnum<vi>)  [unwired: 1 in, 8 out]
            n154 = call "WindowsBoundsToRect.vi"("Windows Bounds"=w395) -> ("Rectangle"=w403:T17)  [unwired: 10 out]
            n155 = call "Calculate Center.vi"("Rectangle"=w401) -> ("Center"=w399:cluster{"x":i32, "y":i32})  [unwired: 10 out]
            n156 = call "Divide Rectangle.vi"("Band (50)"=i16 50, "Rectangle"=w403) -> ("Zones Rectangles"=w400:T18)  [unwired: 1 in, 8 out]
            n157 = for {
              tunnel: w400 -> [w418] mode=indexing
              tunnel: w399 -> [w417]
              tunnel: [w411] -> w398 mode=indexing
              n158 = call "Calculate Center.vi"("Rectangle"=w418) -> ("Center"=w416:cluster{"x":i32, "y":i32})  [unwired: 10 out]
              n159 = Subtract(x=w417, y=w416) -> (x-y=w415:cluster{"x":i32, "y":i32})
              n160 = Absolute Value(x=w415) -> (abs(x)=w414:cluster{"x":i32, "y":i32})
              n161 = Unbundle(w414) -> ("x"=w413:i32, "y"=w412:i32)
              n162 = Add(x=w413, y=w412) -> (x+y=w411:i32)
            }
            n163 = Array Max & Min(array=w398) -> (min index (indices)=w397:i32)  [unwired: 3 out]
            n164 = case shown="1, 4, 6" w397 {
              tunnel: w396 -> [_ w419 w432 w447 w452]
              tunnel: w403 -> [_ w426 w430 w445 w454]
              tunnel: w401 -> [_ w425 w431 w446 w455]
              frame Default {
              }
              frame 1, 4, 6 {
                # "Compensate for Toolbar Border"
                # "Move"
                # "Calculate snapped position"
                n165 = call "Snap to left.vi"("Fixed Rect"=w426, "Rect"=w425) -> ("Snapped to left"=w427:T17)  [unwired: 1 in, 8 out]
                n166 = call "Calculate Center.vi"("Rectangle"=w427) -> ("Center"=w421:cluster{"x":i32, "y":i32})  [unwired: 10 out]
                n167 = Unbundle By Name(w421) -> ("x"=w424:i32)
                n168 = Add(x=w424, y=5) -> (x+y=w422:i32)
                n169 = Bundle By Name(cluster=w421, "x"=w422) -> (w420:cluster{"x":i32, "y":i32})
                n170 = call "MoveObjectonFP.vi"("Move Speed (Instantaneous)"=Move_Speed."Normal", "Center Position for Object"=w420, "GObject"=w419) -> ()  [unwired: 3 in, 6 out]
              }
              frame 2 {
                # "Compensate for Toolbar Border"
                # "Move"
                # "Calculate snapped position"
                n171 = call "Snap to top.vi"("Fixed Rect"=w430, "Rect"=w431) -> ("Snapped to top"=w429:T17)  [unwired: 1 in, 8 out]
                n172 = call "Calculate Center.vi"("Rectangle"=w429) -> ("Center"=w434:cluster{"x":i32, "y":i32})  [unwired: 10 out]
                n173 = Unbundle By Name(w434) -> ("y"=w437:i32)
                n174 = Add(x=w437, y=5) -> (x+y=w435:i32)
                n175 = Bundle By Name(cluster=w434, "y"=w435) -> (w433:cluster{"x":i32, "y":i32})
                n176 = call "MoveObjectonFP.vi"("Move Speed (Instantaneous)"=Move_Speed."Normal", "Center Position for Object"=w433, "GObject"=w432) -> ()  [unwired: 3 in, 6 out]
              }
              frame 3, 5, 8 {
                # "Compensate for Toolbar Border"
                # "Move"
                # "Calculate snapped position"
                n177 = call "Snap to right.vi"("Fixed Rect"=w445, "Rect"=w446) -> ("Snapped to right"=w444:T17)  [unwired: 1 in, 8 out]
                n178 = call "Calculate Center.vi"("Rectangle"=w444) -> ("Center"=w440:cluster{"x":i32, "y":i32})  [unwired: 10 out]
                n179 = Unbundle By Name(w440) -> ("x"=w443:i32)
                n180 = Add(x=w443, y=5) -> (x+y=w441:i32)
                n181 = Bundle By Name(cluster=w440, "x"=w441) -> (w439:cluster{"x":i32, "y":i32})
                n182 = call "MoveObjectonFP.vi"("Move Speed (Instantaneous)"=Move_Speed."Normal", "Center Position for Object"=w439, "GObject"=w447) -> ()  [unwired: 3 in, 6 out]
              }
              frame 7 {
                # "Compensate for Toolbar Border"
                # "Move"
                # "Calculate snapped position"
                n183 = call "Snap to bottom.vi"("Fixed Rect"=w454, "Rect"=w455) -> ("Snapped to bottom"=w453:T17)  [unwired: 1 in, 8 out]
                n184 = call "Calculate Center.vi"("Rectangle"=w453) -> ("Center"=w450:cluster{"x":i32, "y":i32})  [unwired: 10 out]
                n185 = Unbundle By Name(w450) -> ("y"=w457:i32)
                n186 = Add(x=w457, y=5) -> (x+y=w456:i32)
                n187 = Bundle By Name(cluster=w450, "y"=w456) -> (w449:cluster{"x":i32, "y":i32})
                n188 = call "MoveObjectonFP.vi"("Move Speed (Instantaneous)"=Move_Speed."Normal", "Center Position for Object"=w449, "GObject"=w452) -> ()  [unwired: 3 in, 6 out]
              }
            }
            n189 = call <vilib>:"Add State(s) to Queue__JKI_lib_State_Machine.vi"("State(s) in (\"\")"=w409) -> ("States Out"=w408:string)  [unwired: 14 in]
          }
          event Mouse Leave {
            # "Find Closest border"
            n190 = event-data() -> ("CtlRef"=w463:refnum<vi>)  [unwired: 1 in, 3 out]
            n191 = property class="VI"() -> ("Front Panel.PanelBounds"=w467:T16)  [unwired: 2 in, 2 out]
            n192 = call "Calculate_GObject_Rectangle.vi"("GObject ref"=w463) -> ("Rectangle"=w472:T17, "GObject ref dup"=w475:refnum<vi>)  [unwired: 1 in, 8 out]
            n193 = call "WindowsBoundsToRect.vi"("Windows Bounds"=w467) -> ("Rectangle"=w474:T17)  [unwired: 10 out]
            n194 = call "Calculate Center.vi"("Rectangle"=w472) -> ("Center"=w470:cluster{"x":i32, "y":i32})  [unwired: 10 out]
            n195 = call "Divide Rectangle.vi"("Band (50)"=i16 100, "Rectangle"=w474) -> ("Zones Rectangles"=w471:T18)  [unwired: 1 in, 8 out]
            n196 = for {
              tunnel: w471 -> [w483] mode=indexing
              tunnel: w470 -> [w482]
              tunnel: [w476] -> w469 mode=indexing
              n197 = call "Calculate Center.vi"("Rectangle"=w483) -> ("Center"=w481:cluster{"x":i32, "y":i32})  [unwired: 10 out]
              n198 = Subtract(x=w482, y=w481) -> (x-y=w480:cluster{"x":i32, "y":i32})
              n199 = Absolute Value(x=w480) -> (abs(x)=w479:cluster{"x":i32, "y":i32})
              n200 = Unbundle(w479) -> ("x"=w478:i32, "y"=w477:i32)
              n201 = Add(x=w478, y=w477) -> (x+y=w476:i32)
            }
            n202 = Array Max & Min(array=w469) -> (min index (indices)=w468:i32)  [unwired: 3 out]
            n203 = case shown="3, 5, 8" w468 {
              tunnel: w475 -> [_ w488 w505 w518 w530]
              tunnel: w474 -> [_ w495 w499 w523 w534]
              tunnel: w472 -> [_ w494 w500 w524 w535]
              frame Default {
              }
              frame 1, 4, 6 {
                # "Compensate for Toolbar Border"
                # "Move"
                n204 = property class="GObj"(reference=w488) -> (reference out=w487:refnum<vi>, "Bounds"=w489:T19)  [unwired: 1 in, 1 out]
                n205 = Unbundle By Name(w489) -> ("Width"=w486:u32)
                n206 = call "Snap to left.vi"("Fixed Rect"=w495, "Rect"=w494) -> ("Snapped to left"=w496:T17)  [unwired: 1 in, 8 out]
                n207 = call "Calculate Center.vi"("Rectangle"=w496) -> ("Center"=w491:cluster{"x":i32, "y":i32})  [unwired: 10 out]
                n208 = Unbundle By Name(w491) -> ("x"=w493:i32)
                n209 = Subtract(x=w486, y=u32 5) -> (x-y=w484:u32)
                n210 = Subtract(x=w493, y=w484) -> (x-y=w492:u32)
                n211 = Bundle By Name(cluster=w491, "x"=w492) -> (w490:cluster{"x":i32, "y":i32})
                n212 = call "MoveObjectonFP.vi"("Move Speed (Instantaneous)"=Move_Speed."Normal", "Center Position for Object"=w490, "GObject"=w487) -> ()  [unwired: 3 in, 6 out]
              }
              frame 2 {
                # "Compensate for Toolbar Border"
                # "Move"
                # "Calculate snapped position"
                n213 = property class="GObj"(reference=w505) -> (reference out=w504:refnum<vi>, "Bounds"=w506:T19)  [unwired: 1 in, 1 out]
                n214 = Unbundle By Name(w506) -> ("Height"=w503:u32)
                n215 = call "Snap to top.vi"("Fixed Rect"=w499, "Rect"=w500) -> ("Snapped to top"=w498:T17)  [unwired: 1 in, 8 out]
                n216 = call "Calculate Center.vi"("Rectangle"=w498) -> ("Center"=w508:cluster{"x":i32, "y":i32})  [unwired: 10 out]
                n217 = Unbundle By Name(w508) -> ("y"=w510:i32)
                n218 = Subtract(x=w503, y=u32 5) -> (x-y=w501:u32)
                n219 = Subtract(x=w510, y=w501) -> (x-y=w509:u32)
                n220 = Bundle By Name(cluster=w508, "y"=w509) -> (w507:cluster{"x":i32, "y":i32})
                n221 = call "MoveObjectonFP.vi"("Move Speed (Instantaneous)"=Move_Speed."Normal", "Center Position for Object"=w507, "GObject"=w504) -> ()  [unwired: 3 in, 6 out]
              }
              frame 3, 5, 8 {
                # "Compensate for Toolbar Border"
                # "Move"
                n222 = property class="GObj"(reference=w518) -> (reference out=w517:refnum<vi>, "Bounds"=w519:T19)  [unwired: 1 in, 1 out]
                n223 = Unbundle By Name(w519) -> ("Width"=w514:u32)
                n224 = call "Snap to right.vi"("Fixed Rect"=w523, "Rect"=w524) -> ("Snapped to right"=w522:T17)  [unwired: 1 in, 8 out]
                n225 = call "Calculate Center.vi"("Rectangle"=w522) -> ("Center"=w521:cluster{"x":i32, "y":i32})  [unwired: 10 out]
                n226 = Add(x=w514, y=5) -> (x+y=w512:u32)
                n227 = Unbundle By Name(w521) -> ("x"=w516:i32)
                n228 = Add(x=w512, y=w516) -> (x+y=w515:u32)
                n229 = Bundle By Name(cluster=w521, "x"=w515) -> (w520:cluster{"x":i32, "y":i32})
                n230 = call "MoveObjectonFP.vi"("Move Speed (Instantaneous)"=Move_Speed."Normal", "Center Position for Object"=w520, "GObject"=w517) -> ()  [unwired: 3 in, 6 out]
              }
              frame 7 {
                # "Compensate for Toolbar Border"
                # "Move"
                n231 = call "Snap to bottom.vi"("Fixed Rect"=w534, "Rect"=w535) -> ("Snapped to bottom"=w533:T17)  [unwired: 1 in, 8 out]
                n232 = property class="GObj"(reference=w530) -> (reference out=w529:refnum<vi>, "Height"=w532:u32)  [unwired: 1 in, 1 out]
                n233 = call "Calculate Center.vi"("Rectangle"=w533) -> ("Center"=w537:cluster{"x":i32, "y":i32})  [unwired: 10 out]
                n234 = Unbundle By Name(w537) -> ("y"=w527:i32)
                n235 = Add(x=w532, y=u32 5) -> (x+y=w526:u32)
                n236 = Add(x=w527, y=w526) -> (x+y=w528:u32)
                n237 = Bundle By Name(cluster=w537, "y"=w528) -> (w536:cluster{"x":i32, "y":i32})
                n238 = call "MoveObjectonFP.vi"("Move Speed (Instantaneous)"=Move_Speed."Normal", "Center Position for Object"=w536, "GObject"=w529) -> ()  [unwired: 3 in, 6 out]
              }
            }
            n239 = call <vilib>:"Add State(s) to Queue__JKI_lib_State_Machine.vi"("State(s) in (\"\")"=w464) -> ("States Out"=w465:string)  [unwired: 14 in]
          }
          event "TOP10_返回": Mouse Down {
            n240 = event-data() -> ()  [unwired: 1 in, 8 out]
            n241 = local write "选项卡控件"(选项卡枚举."主界面" ("枚举")) -> ()
            n242 = call <vilib>:"Add State(s) to Queue__JKI_lib_State_Machine.vi"("State(s) in (\"\")"=w546, "State(s) at Back (\"\")"="UI: Initialize" ("State(s) at Back (\"\")")) -> ("States Out"=w545:string)  [unwired: 13 in]
          }
          event Key Down {
            n243 = event-data() -> ("VKey"=w550:T20)  [unwired: 1 in, 3 out]
            n244 = local read "键盘启用"() -> (w549:bool)
            n245 = case shown="真" w549 {
              tunnel: ["Idle" ("State(s) at Back (\"\")") w563] -> w555
              tunnel: [w559 w562] -> w554
              tunnel: w550 -> [_ w561]
              tunnel: w548 -> [w559 _]
              frame False {
              }
              frame True {
                n246 = case shown="\"Left\"" w561 {
                  tunnel: [按键枚举."退出" 按键枚举."绿" 按键枚举."蓝" 按键枚举."红" 按键枚举."黄"] -> w562
                  tunnel: ["Idle" ("State(s) at Back (\"\")") "Game: Option" ("State(s) at Back (\"\")") "Game: Option" ("State(s) at Back (\"\")") "Game: Option" ("State(s) at Back (\"\")") "Game: Option" ("State(s) at Back (\"\")")] -> w563
                  frame "ASCII", Default {
                  }
                  frame "Up" {
                    n247 = stacked-sequence {
                      frame #0 {
                        n248 = local write "游戏界面_上"(TRUE ("上")) -> ()
                      }
                      frame #1 {
                        n249 = Wait (ms)(milliseconds to wait=u32 60 ("等待时间（毫秒）")) -> ()  [unwired: 1 out]
                      }
                      frame #2 {
                        n250 = local write "游戏界面_上"(FALSE ("上")) -> ()
                      }
                      frame #3 {
                        n251 = Wait (ms)(milliseconds to wait=u32 60 ("等待时间（毫秒）")) -> ()  [unwired: 1 out]
                      }
                    }
                  }
                  frame "Right" {
                    n252 = stacked-sequence {
                      frame #0 {
                        n253 = local write "游戏界面_右"(TRUE ("上")) -> ()
                      }
                      frame #1 {
                        n254 = Wait (ms)(milliseconds to wait=u32 60 ("等待时间（毫秒）")) -> ()  [unwired: 1 out]
                      }
                      frame #2 {
                        n255 = local write "游戏界面_右"(FALSE ("上")) -> ()
                      }
                      frame #3 {
                        n256 = Wait (ms)(milliseconds to wait=u32 60 ("等待时间（毫秒）")) -> ()  [unwired: 1 out]
                      }
                    }
                  }
                  frame "Down" {
                    n257 = stacked-sequence {
                      frame #0 {
                        n258 = local write "游戏界面_下"(TRUE ("上")) -> ()
                      }
                      frame #1 {
                        n259 = Wait (ms)(milliseconds to wait=u32 60 ("等待时间（毫秒）")) -> ()  [unwired: 1 out]
                      }
                      frame #2 {
                        n260 = local write "游戏界面_下"(FALSE ("上")) -> ()
                      }
                      frame #3 {
                        n261 = Wait (ms)(milliseconds to wait=u32 60 ("等待时间（毫秒）")) -> ()  [unwired: 1 out]
                      }
                    }
                  }
                  frame "Left" {
                    n262 = stacked-sequence {
                      frame #0 {
                        n263 = local write "游戏界面_左"(TRUE ("上")) -> ()
                      }
                      frame #1 {
                        n264 = Wait (ms)(milliseconds to wait=u32 60 ("等待时间（毫秒）")) -> ()  [unwired: 1 out]
                      }
                      frame #2 {
                        n265 = local write "游戏界面_左"(FALSE ("上")) -> ()
                      }
                      frame #3 {
                        n266 = Wait (ms)(milliseconds to wait=u32 60 ("等待时间（毫秒）")) -> ()  [unwired: 1 out]
                      }
                    }
                  }
                }
              }
            }
            n267 = call <vilib>:"Add State(s) to Queue__JKI_lib_State_Machine.vi"("State(s) in (\"\")"=w556, "State(s) at Back (\"\")"=w555) -> ("States Out"=w557:string)  [unwired: 13 in]
          }
          event "游戏规则_返回": Mouse Down {
            n268 = event-data() -> ()  [unwired: 1 in, 8 out]
            n269 = local write "选项卡控件"(选项卡枚举."主界面" ("枚举")) -> ()
            n270 = call <vilib>:"Add State(s) to Queue__JKI_lib_State_Machine.vi"("State(s) in (\"\")"=w596, "State(s) at Back (\"\")"="UI: Initialize" ("State(s) at Back (\"\")")) -> ("States Out"=w597:string)  [unwired: 13 in]
          }
          event "TOP10_退出": Value Change {
            # "Exit Button Value Change (pressed) Event\n(this executes Macro: Exit to terminate the VI)"
            n271 = event-data() -> ()  [unwired: 1 in, 1 out]
            n272 = local write "是否开始计时？"(FALSE ("是否开始计时？")) -> ()
            n273 = call <vilib>:"Add State(s) to Queue__JKI_lib_State_Machine.vi"("State(s) in Front (\"\")"="Macro: Exit", "State(s) in (\"\")"=w607) -> ("States Out"=w606:string)  [unwired: 13 in]
          }
          event Panel Close? {
            # "Discard the event because we'll close the front panel ourselves in Macro: Exit"
            # "Close Panel button (pressed) Event\n(this executes Macro: Exit to terminate the VI)"
            n274 = event-data() -> ()  [unwired: 1 in, 1 out]
            n275 = call <vilib>:"Add State(s) to Queue__JKI_lib_State_Machine.vi"("State(s) in Front (\"\")"="Macro: Exit", "State(s) in (\"\")"=w616) -> ("States Out"=w615:string)  [unwired: 13 in]
            n276 = event-data("Discard?"=TRUE) -> ()  [unwired: 1 in, 1 out]
          }
        }
      }
      frame "---------- Core ----------" {
        # "Do not put any code in this frame.\n(it is a separator no-op)"
        n277 = call <vilib>:"Add State(s) to Queue__JKI_lib_State_Machine.vi"("State(s) in (\"\")"=w623) -> ("States Out"=w622:string)  [unwired: 14 in]
      }
      frame Default {
        w636 = 42 items=["No error", "Argument error", "Memory is full", "Out of zone", "End of file", "File already open", "Generic file I/O error", "File not found", "File permission error", "Disk is full", "Duplicate path", "Too many files open", "System feature not enabled", "Resource file not found", "Cannot add resource", "Resource not found", "Image not found", "Image memory error", "Pen does not exist", "Config type invalid", "Config token not found", "Config parse error", "Config memory error", "Bad external code format", "Bad external code offset", "External code not present", "Null window", "Destroy window error", "Null menu", "Print aborted", "Bad print record", "Print driver error", "Windows error during printing", "Memory error during printing", "Print dialog error", "Generic print error", "Invalid device refnum", "Device not found", "Device parameter error", "Device unit error", "Cannot open device", "Device call aborted", "Generic error", "Cancelled by user", "Object ID too low", "Object ID too high", "Object not in heap", "Unknown heap", "Unknown object (invalid DefProc)", "Unknown object (DefProc not in table)", "Message out of range", "Invalid (null) method", "Unknown message", "Manager call not supported", "Bad address", "Network operation in progress", "Network operation timed out", "Connection is busy", "Network attribute not supported", "Network error", "Address in use", "System out of memory", "Connection aborted", "Connection refused", "Not connected", "Already connected", "Connection closed", "Initialization error (interapplication manager)", "Bad occurrence", "Wait on unbound occurrence handler", "Occurrence queue overflow", "Datalog type conflict", "Unused", "Unrecognized type (interapplication manager)", "Memory corrupt", "Failed to make temporary DLL", "Old CIN version", "Drag socket not found", "Failed to load drop-object", "Failed to register OLE object", "Failed to release OLE object", "Format specifier type mismatch", "Unknown format specifier", "Too few format specifiers", "Too many format specifiers", "Scan failed", "Newer CIN version", "Error converting to variant", "Runtime menu error", "Password tampered", "Variant attribute not found", "Incompatible variant data type", "Event data is not available", "Event Store is not present", "Occurrence is not found", "Event Queue is not created", "Event info is not available", "Refnum passed is NULL", "Error retrieving Class GUID", "Error retrieving CoClass GUID", "Error retrieving TypeLib GUID.", "Bad built application magic bytes.", "Specific driver is different from the specific driver associated with the Logical Name.", "There is no session opened to the class driver.", "Max Error", "MAX - Error with config objects", "MAX - Error loading configuration", "MAX - Group not supported"]
        # "Current State"
        # "Do not delete, rename, or modify this frame.\n(this is used to capture unhandled states and typos)"
        # "Handle mistyped state name (developer tool)"
        n278 = Format Into String(format string="Software Exception: Unhandled State \"%s\"." ("message"), error in=w632, w627) -> (resulting string=w635:string, error out=w634:errorcluster)  [unwired: 1 in]
        n279 = call <vilib>:"Error Cluster From Error Code.vi"("show call chain? (False)"=TRUE, "error in (no error)"=w634, "error message (\"\")"=w635, "error code (0)"=w636) -> ("error out"=w633:errorcluster)  [unwired: 5 in]
        n280 = call <vilib>:"Add State(s) to Queue__JKI_lib_State_Machine.vi"("State(s) in (\"\")"=w631) -> ("States Out"=w630:string)  [unwired: 14 in]
      }
      frame "Initialize Core Data" {
        # "Do not delete, rename, or modify this frame.\n(this is used to determine panel behavior on exit)"
        # "originally closed?"
        # "exe?"
        # "If panel starts closed or is an EXE, then close it when we exit"
        n281 = property class="VI"() -> ("FP.State"=w643:T13)  [unwired: 2 in, 2 out]
        n282 = control-ref of="Current VI Reference"() -> (w644:refnum<vi>)
        n283 = Equal?(x=w643, y=T13."Closed" ("Front Panel Window:State")) -> (x = y?=w641:bool)
        n284 = property class="App"() -> ("App.Kind"=w649:T14)  [unwired: 2 in, 2 out]
        n285 = Equal?(x=w649, y=T14."Run Time System" ("Application:Kind")) -> (x = y?=w647:bool)
        n286 = Or(x=w641, y=w647) -> (x .or. y?=w645:bool)
        n287 = Bundle By Name(cluster=w646, "Core.Current VI Reference"=w644, "Core.Close Panel on Exit?"=w645) -> (w651:T15)
        n288 = call <vilib>:"Add State(s) to Queue__JKI_lib_State_Machine.vi"("State(s) in (\"\")"=w653) -> ("States Out"=w652:string)  [unwired: 14 in]
      }
      frame "Error Handler" {
        # "Unhandled Error -- Display it"
        # "Handle any errors here.\nYou can also output any states to clean-up after errors occur"
        # "Clear error"
        n289 = call <vilib>:"General Error Handler.vi"("error in (no error)"=w658) -> ()  [unwired: 10 in, 5 out]
        n290 = call <vilib>:"Add State(s) to Queue__JKI_lib_State_Machine.vi"("State(s) in Front (\"\")"="/* Post Error States", "State(s) in (\"\")"=w662) -> ("States Out"=w661:string)  [unwired: 13 in]
      }
      frame "Exit" {
        # "Do not put any code in this frame.\n(No errors that occur here will be handled.)"
        n291 = call <vilib>:"Add State(s) to Queue__JKI_lib_State_Machine.vi"("State(s) in (\"\")"=w670) -> ("States Out"=w669:string)  [unwired: 14 in]
      }
      frame "---------- Data ----------" {
        # "Do not put any code in this frame.\n(It is a separator no-op. You can make a copy of this frame to create a new Data frame)"
        n292 = call <vilib>:"Add State(s) to Queue__JKI_lib_State_Machine.vi"("State(s) in (\"\")"=w677) -> ("States Out"=w676:string)  [unwired: 14 in]
      }
      frame "Data: Initialize" {
        w683 = 0  # 积分_排名
        w691 = ""  # 难度_保存
        w687 = 0  # 积分_保存
        w688 = 0  # 闪烁间隔_保存
        w689 = 0  # 超时时间_保存
        w690 = 0  # 亮灯次数_保存
        w692 = ""  # 用户名
        w693 = ""  # 修改密码_账户
        w694 = ""  # 修改密码_新密码
        w695 = ""  # 注册密码
        w696 = T21 {"Current VI Reference"=refnum, "Close Panel on Exit?"=FALSE}  # Core
        w698 = TRUE  # Your Boolean data
        w697 = ""  # 注册账户
        # "do not delete - used by framework"
        # "Add new data here."
        # "Initialize the shift-register data, here.\n(data names are defined by what you wire into the bundle function)"
        n293 = invoke on="选项卡控件" class="TabCtl (严格)" method="Reinit To Default"() -> ()  [unwired: 3 in, 3 out]
        n294 = property on="玩家                      积分          简单" class="Arr (严格)"("Index Visible"=FALSE ("索引可见")) -> ()  [unwired: 2 in, 2 out]
        n295 = property on="玩家                      积分          困难" class="Arr (严格)"("Index Visible"=FALSE ("索引可见")) -> ()  [unwired: 2 in, 2 out]
        n296 = property on="玩家                      积分          中等" class="Arr (严格)"("Index Visible"=FALSE ("索引可见")) -> ()  [unwired: 2 in, 2 out]
        n297 = property on="Toolbar 5" class="Clust (严格)"("Visible"=FALSE ("可见")) -> ()  [unwired: 2 in, 2 out]
        n298 = property on="AniGIF" class="AXCont"("Visible"=TRUE ("可见")) -> ()  [unwired: 2 in, 2 out]
        n299 = Bundle("Core"=w696, "Your Boolean data"=w698, "注册账户"=w697, "注册密码"=w695, "修改密码_新密码"=w694, "修改密码_账户"=w693, "用户名"=w692, "难度_保存"=w691, "亮灯次数_保存"=w690, "超时时间_保存"=w689, "闪烁间隔_保存"=w688, "积分_保存"=w687, "积分_排名"=w683) -> (w700:T15)  [unwired: 1 in]
        n300 = call <vilib>:"Add State(s) to Queue__JKI_lib_State_Machine.vi"("State(s) in (\"\")"=w702) -> ("States Out"=w701:string)  [unwired: 14 in]
      }
      frame "Data: Cleanup" {
        # "Cleanup any data and references, here.\n(this is called automatically, by the Macro: Exit)"
        n301 = Unbundle By Name(w706) -> ("Core.Current VI Reference"=w709:refnum<vi>)
        n302 = Close Reference(reference=w709, error in (no error)=w708) -> (error out=w707:errorcluster)
        n303 = call <vilib>:"Add State(s) to Queue__JKI_lib_State_Machine.vi"("State(s) in (\"\")"=w711) -> ("States Out"=w710:string)  [unwired: 14 in]
      }
      frame "---------- UI ----------" {
        # "Do not put any code in this frame.\n(It is a separator no-op. You can make a copy of this frame to create a new UI frame)"
        n304 = call <vilib>:"Add State(s) to Queue__JKI_lib_State_Machine.vi"("State(s) in (\"\")"=w718) -> ("States Out"=w717:string)  [unwired: 14 in]
      }
      frame "UI: Initialize" {
        # "Initialize the User Interface, here.\n(this is called automatically, by the Macro: Init)"
        n305 = invoke on="密码:" class="Str" method="Reinit To Default"() -> ()  [unwired: 3 in, 3 out]
        n306 = invoke on="账号:" class="Str" method="Reinit To Default"() -> ()  [unwired: 3 in, 3 out]
        n307 = invoke on="用户注册_返回" class="Bool (严格)" method="Reinit To Default"() -> ()  [unwired: 3 in, 3 out]
        n308 = invoke on="用户注册_注册" class="Bool (严格)" method="Reinit To Default"() -> ()  [unwired: 3 in, 3 out]
        n309 = invoke on="是否开始计时？" class="Bool (严格)" method="Reinit To Default"() -> ()  [unwired: 3 in, 3 out]
        n310 = invoke on="游戏界面_读档" class="Bool (严格)" method="Reinit To Default"() -> ()  [unwired: 3 in, 3 out]
        n311 = invoke on="游戏界面_存档" class="Bool (严格)" method="Reinit To Default"() -> ()  [unwired: 3 in, 3 out]
        n312 = invoke on="游戏界面_结束" class="Bool (严格)" method="Reinit To Default"() -> ()  [unwired: 3 in, 3 out]
        n313 = invoke on="调用节点" class="IAniGIF" method="Play"(reference="AniGIF") -> ()  [unwired: 2 in, 3 out]
        n314 = invoke on="修改密码_修改" class="Bool (严格)" method="Reinit To Default"() -> ()  [unwired: 3 in, 3 out]
        n315 = invoke on="修改密码_返回" class="Bool (严格)" method="Reinit To Default"() -> ()  [unwired: 3 in, 3 out]
        n316 = invoke on="主界面_进入游戏" class="Bool (严格)" method="Reinit To Default"() -> ()  [unwired: 3 in, 3 out]
        n317 = invoke on="主界面_返回" class="Bool (严格)" method="Reinit To Default"() -> ()  [unwired: 3 in, 3 out]
        n318 = invoke on="主界面_TOP10" class="Bool (严格)" method="Reinit To Default"() -> ()  [unwired: 3 in, 3 out]
        n319 = property on="选项卡控件" class="TabCtl (严格)"("PageSelVis"=FALSE ("选项卡标签显示可见？")) -> ()  [unwired: 2 in, 2 out]
        n320 = invoke on="主界面_游戏规则" class="Bool (严格)" method="Reinit To Default"() -> ()  [unwired: 3 in, 3 out]
        n321 = invoke on="登录界面_登录" class="Bool (严格)" method="Reinit To Default"() -> ()  [unwired: 3 in, 3 out]
        n322 = invoke on="登录界面_退出" class="Bool (严格)" method="Reinit To Default"() -> ()  [unwired: 3 in, 3 out]
        n323 = invoke on="登陆界面_注册" class="Bool (严格)" method="Reinit To Default"() -> ()  [unwired: 3 in, 3 out]
        n324 = invoke on="登录界面_修改密码" class="Bool (严格)" method="Reinit To Default"() -> ()  [unwired: 3 in, 3 out]
        n325 = invoke on="键盘启用" class="Bool (严格)" method="Reinit To Default"() -> ()  [unwired: 3 in, 3 out]
        n326 = invoke on="游戏规则_返回" class="Bool (严格)" method="Reinit To Default"() -> ()  [unwired: 3 in, 3 out]
        n327 = call <vilib>:"Application Directory.vi"() -> ("Application Directory"=w726:path)
        n328 = invoke on="注册密码:" class="Str" method="Reinit To Default"() -> ()  [unwired: 3 in, 3 out]
        n329 = invoke on="确认密码:" class="Str" method="Reinit To Default"() -> ()  [unwired: 3 in, 3 out]
        n330 = invoke on="注册账户:" class="Str" method="Reinit To Default"() -> ()  [unwired: 3 in, 3 out]
        n331 = invoke on="TOP10_返回" class="Bool (严格)" method="Reinit To Default"() -> ()  [unwired: 3 in, 3 out]
        n332 = invoke on="TOP10_退出" class="Bool (严格)" method="Reinit To Default"() -> ()  [unwired: 3 in, 3 out]
        n333 = invoke on="账号:" class="Str" method="Reinit To Default"() -> ()  [unwired: 3 in, 3 out]
        n334 = invoke on="确认密码:" class="Str" method="Reinit To Default"() -> ()  [unwired: 3 in, 3 out]
        n335 = invoke on="旧密码:" class="Str" method="Reinit To Default"() -> ()  [unwired: 3 in, 3 out]
        n336 = invoke on="新密码:" class="Str" method="Reinit To Default"() -> ()  [unwired: 3 in, 3 out]
        n337 = Build Path(base path=w726, name or relative path="排名简单.txt" ("名称或相对路径")) -> (appended path=w729:path)
        n338 = Build Path(base path=w726, name or relative path="排名中等.txt" ("名称或相对路径")) -> (appended path=w728:path)
        n339 = Build Path(base path=w726, name or relative path="排名困难.txt" ("名称或相对路径")) -> (appended path=w727:path)
        n340 = call-poly <vilib>:"Read Delimited Spreadsheet.vi"("file path (dialog if empty)"=w729) -> ("all rows"=w723:string[][])  [unwired: 9 in, 5 out]
        n341 = call-poly <vilib>:"Read Delimited Spreadsheet.vi"("file path (dialog if empty)"=w728) -> ("all rows"=w724:string[][])  [unwired: 9 in, 5 out]
        n342 = call-poly <vilib>:"Read Delimited Spreadsheet.vi"("file path (dialog if empty)"=w727) -> ("all rows"=w725:string[][])  [unwired: 9 in, 5 out]
        n343 = invoke on="键盘启用" class="Bool (严格)" method="Reinit To Default"() -> ()  [unwired: 3 in, 3 out]
        n344 = invoke on="游戏界面_时间到" class="Bool (严格)" method="Reinit To Default"() -> ()  [unwired: 3 in, 3 out]
        n345 = local write "玩家                      积分          中等"(w724) -> ()
        n346 = local write "玩家                      积分          简单"(w723) -> ()
        n347 = local write "玩家                      积分          困难"(w725) -> ()
        n348 = invoke on="亮灯次数" class="DigNum (严格)" method="Reinit To Default"() -> ()  [unwired: 3 in, 3 out]
        n349 = invoke on="分数" class="DigNum (严格)" method="Reinit To Default"() -> ()  [unwired: 3 in, 3 out]
        n350 = invoke on="难度：分数" class="Str" method="Reinit To Default"() -> ()  [unwired: 3 in, 3 out]
        n351 = property on="TOP10_返回" class="Bool (严格)"("Visible"=TRUE ("可见")) -> ()  [unwired: 2 in, 2 out]
        n352 = property on="TOP10_退出" class="Bool (严格)"("Visible"=FALSE ("可见")) -> ()  [unwired: 2 in, 2 out]
        n353 = call <vilib>:"Add State(s) to Queue__JKI_lib_State_Machine.vi"("State(s) in (\"\")"=w739) -> ("States Out"=w738:string)  [unwired: 14 in]
      }
      frame "UI: Cursor Set" {
        # "Argument"
        # "Set and Unset Cursor Busy.\n(Usage: \"UI: Cursor Set >> Busy|Idle\")"
        n354 = case shown="\"Idle\", 默认" w743 {
          tunnel: w745 -> [w750 w752]
          tunnel: [w749 w751] -> w744
          frame "Idle", Default {
            n355 = call <vilib>:"Unset Busy.vi"("error in (no error)"=w750) -> ("error out"=w749:errorcluster)  [unwired: 10 in]
          }
          frame "Busy" {
            n356 = call <vilib>:"Set Busy.vi"("error in (no error)"=w752) -> ("error out"=w751:errorcluster)  [unwired: 9 in, 1 out]
          }
        }
        n357 = call <vilib>:"Add State(s) to Queue__JKI_lib_State_Machine.vi"("State(s) in (\"\")"=w748) -> ("States Out"=w747:string)  [unwired: 14 in]
      }
      frame "UI: Front Panel State" {
        # "Argument"
        # "Set Front Panel Open or Closed\n(Usage: \"UI: Front Panel State >> Open|Close\")"
        n358 = Unbundle By Name(w758) -> ("Core.Current VI Reference"=w757:refnum<vi>)
        n359 = case shown="\"Open\", \"Standard\", 默认" w756 {
          tunnel: w760 -> [w768 w783 w794 w807 w820]
          tunnel: [w770 w784 w796 w809 w822] -> w759
          tunnel: w757 -> [w769 w781 w795 w808 w821]
          frame "Open", "Standard", Default {
            w763 = T13."Standard" ("State")
            n360 = property class="VI"(reference=w769, error in=w768) -> (reference out=w766:refnum<vi>, error out=w767:errorcluster, "FP.State"=w765:T13)
            n361 = Not Equal?(x=w765, y=w763) -> (x != y?=w764:bool)
            n362 = case shown="假" w764 {
              tunnel: [w774 w776] -> w770
              tunnel: w767 -> [w773 w776]
              tunnel: w766 -> [w772 _]
              tunnel: w763 -> [w771 _]
              frame True {
                n363 = invoke class="VI" method="FP.Open"(reference=w772, error in=w773, "Activate"=TRUE, "State"=w771) -> (error out=w774:errorcluster)  [unwired: 1 in, 4 out]
              }
              frame False {
              }
            }
          }
          frame "Close", "Closed" {
            n364 = property class="VI"(reference=w781, error in=w783) -> (reference out=w780:refnum<vi>, error out=w782:errorcluster, "FP.State"=w778:T13)
            n365 = Not Equal?(x=w778, y=T13."Closed" ("Front Panel Window:State")) -> (x != y?=w777:bool)
            n366 = case shown="真" w777 {
              tunnel: [w785 w788] -> w784
              tunnel: w782 -> [w785 w787]
              tunnel: w780 -> [_ w786]
              frame False {
              }
              frame True {
                n367 = invoke class="VI" method="FP.Close"(reference=w786, error in=w787) -> (error out=w788:errorcluster)  [unwired: 1 in, 2 out]
              }
            }
          }
          frame "Hidden", "Hide" {
            w789 = T13."Hidden" ("State")
            n368 = property class="VI"(reference=w795, error in=w794) -> (reference out=w792:refnum<vi>, error out=w793:errorcluster, "FP.State"=w791:T13)
            n369 = Not Equal?(x=w791, y=w789) -> (x != y?=w790:bool)
            n370 = case shown="真" w790 {
              tunnel: [w800 w801] -> w796
              tunnel: w793 -> [w799 w801]
              tunnel: w792 -> [w798 _]
              tunnel: w789 -> [w797 _]
              frame True {
                n371 = invoke class="VI" method="FP.Open"(reference=w798, error in=w799, "State"=w797) -> (error out=w800:errorcluster)  [unwired: 2 in, 4 out]
              }
              frame False {
              }
            }
          }
          frame "Minimize", "Minimized" {
            w802 = T13."Minimized" ("State")
            n372 = property class="VI"(reference=w808, error in=w807) -> (reference out=w805:refnum<vi>, error out=w806:errorcluster, "FP.State"=w804:T13)
            n373 = Not Equal?(x=w804, y=w802) -> (x != y?=w803:bool)
            n374 = case shown="真" w803 {
              tunnel: [w813 w814] -> w809
              tunnel: w806 -> [w812 w814]
              tunnel: w805 -> [w811 _]
              tunnel: w802 -> [w810 _]
              frame True {
                n375 = invoke class="VI" method="FP.Open"(reference=w811, error in=w812, "State"=w810) -> (error out=w813:errorcluster)  [unwired: 2 in, 4 out]
              }
              frame False {
              }
            }
          }
          frame "Maximize", "Maximized" {
            w815 = T13."Maximized" ("State")
            n376 = property class="VI"(reference=w821, error in=w820) -> (reference out=w818:refnum<vi>, error out=w819:errorcluster, "FP.State"=w817:T13)
            n377 = Not Equal?(x=w817, y=w815) -> (x != y?=w816:bool)
            n378 = case shown="真" w816 {
              tunnel: [w826 w827] -> w822
              tunnel: w819 -> [w825 w827]
              tunnel: w818 -> [w824 _]
              tunnel: w815 -> [w823 _]
              frame True {
                n379 = invoke class="VI" method="FP.Open"(reference=w824, error in=w825, "State"=w823) -> (error out=w826:errorcluster)  [unwired: 2 in, 4 out]
              }
              frame False {
              }
            }
          }
        }
        n380 = call <vilib>:"Add State(s) to Queue__JKI_lib_State_Machine.vi"("State(s) in (\"\")"=w762) -> ("States Out"=w761:string)  [unwired: 14 in]
      }
      frame "---------- Macro ----------" {
        # "Do not put any code in this frame.\n(It is a separator no-op. You can make a copy of this frame to create a new Macro frame)"
        n381 = call <vilib>:"Add State(s) to Queue__JKI_lib_State_Machine.vi"("State(s) in (\"\")"=w834) -> ("States Out"=w833:string)  [unwired: 14 in]
      }
      frame "Macro: Initialize" {
        # "Initialization Macro\n(This is called once, when the VI starts)"
        n382 = call <vilib>:"Add State(s) to Queue__JKI_lib_State_Machine.vi"("State(s) in Front (\"\")"="Data: Initialize\nInitialize Core Data\nUI: Initialize\nUI: Front Panel State >> Open", "State(s) in (\"\")"=w842) -> ("States Out"=w841:string)  [unwired: 13 in]
      }
      frame "Macro: Exit" {
        # "Exit Macro\n(This is called once, when the VI exits)"
        n383 = Unbundle By Name(w852) -> ("Core.Close Panel on Exit?"=w851:bool)
        n384 = Select(t="UI: Front Panel State >> Close", s=w851, f="") -> (s? t:f=w848:string)
        n385 = call <vilib>:"Add State(s) to Queue__JKI_lib_State_Machine.vi"("State(s) in (\"\")"=w848, "State(s) at Back (\"\")"="Data: Cleanup\nExit") -> ("States Out"=w846:string)  [unwired: 13 in]
        n386 = call <vilib>:"Add State(s) to Queue__JKI_lib_State_Machine.vi"("State(s) in Front (\"\")"=w846, "State(s) in (\"\")"=w855) -> ("States Out"=w854:string)  [unwired: 13 in]
      }
      frame "---------- User ----------" {
        # "Template Separator\n(You can make a copy of, or modify, this frame)"
        n387 = call <vilib>:"Add State(s) to Queue__JKI_lib_State_Machine.vi"("State(s) in (\"\")"=w862) -> ("States Out"=w861:string)  [unwired: 14 in]
      }
      frame "User: Info" {
        # "Template Separator\n(You can make a copy of, or modify, this frame)"
        n388 = case shown="\"register\"" w866 {
          tunnel: w869 -> [w886 w895]
          tunnel: ["UI: Initialize" "UI: Initialize"] -> w868
          frame "modify", Default {
            # "获取待修改账户的行索引"
            # "获取第0列数组"
            n389 = Unbundle By Name(w886) -> ("修改密码_账户"=w876:string, "修改密码_新密码"=w881:string)
            n390 = call <vilib>:"Application Directory.vi"() -> ("Application Directory"=w888:path)
            n391 = local write "选项卡控件"(选项卡枚举."登录界面" ("枚举")) -> ()
            n392 = Build Array(w876, w881) -> (w880:string[])
            n393 = Build Path(base path=w888, name or relative path="账户信息.txt" ("名称或相对路径")) -> (appended path=w879:path)
            n394 = Concatenate Strings("用户“" ("字符串"), w876, "”密码修改成功" ("字符串")) -> (w874:string)
            n395 = One Button Dialog(message=w874) -> ()  [unwired: 1 in, 1 out]
            n396 = call-poly <vilib>:"Read Delimited Spreadsheet.vi"("file path (dialog if empty)"=w879) -> ("all rows"=w883:string[][])  [unwired: 9 in, 5 out]
            n397 = Index Array(array=w883, index (col)=0 ("禁用的索引 (列)")) -> (element=w884:string[])  [unwired: 1 in]
            n398 = Search 1D Array(1D array=w884, element=w876) -> (index of element=w882:i32)  [unwired: 1 in]
            n399 = Replace Array Subset(array=w883, new element=w880, index (row)=w882) -> (w878:string[][])  [unwired: 1 in]
            n400 = call-poly <vilib>:"Write Delimited Spreadsheet.vi"("file path (dialog if empty)"=w879, "2D data"=w878) -> ()  [unwired: 12 in, 2 out]
          }
          frame "register" {
            n401 = Unbundle By Name(w895) -> ("注册账户"=w894:string, "注册密码"=w893:string)
            n402 = Build Array(w894, w893) -> (w892:string[])
            n403 = call <vilib>:"Application Directory.vi"() -> ("Application Directory"=w899:path)
            n404 = local write "选项卡控件"(选项卡枚举."登录界面" ("枚举")) -> ()
            n405 = Build Path(base path=w899, name or relative path="账户信息.txt" ("名称或相对路径")) -> (appended path=w897:path)
            n406 = call-poly <vilib>:"Write Delimited Spreadsheet.vi"("file path (dialog if empty)"=w897, "1D data"=w892, "append to file? (new file:F)"=TRUE) -> ()  [unwired: 11 in, 2 out]
          }
        }
        n407 = Wait (ms)(milliseconds to wait=u32 50 ("等待时间（毫秒）")) -> ()  [unwired: 1 out]
        n408 = call <vilib>:"Add State(s) to Queue__JKI_lib_State_Machine.vi"("State(s) in (\"\")"=w872, "State(s) at Back (\"\")"=w868) -> ("States Out"=w871:string)  [unwired: 13 in]
      }
      frame "User: login" {
        w913 = 0 ("y")
        # "获取第0列数组"
        # "根据账户索引获取密码"
        # "查询账户，获取账户索引"
        # "Your code here.\n(You can make a copy of, or modify, this frame)"
        n409 = call <vilib>:"Application Directory.vi"() -> ("Application Directory"=w925:path)
        n410 = Build Path(base path=w925, name or relative path="账户信息.txt" ("名称或相对路径")) -> (appended path=w923:path)
        n411 = call-poly <vilib>:"Read Delimited Spreadsheet.vi"("file path (dialog if empty)"=w923) -> ("all rows"=w917:string[][])  [unwired: 9 in, 5 out]
        n412 = Index Array(array=w917, index (col)=0 ("禁用的索引 (列)")) -> (element=w921:string[])  [unwired: 1 in]
        n413 = Search 1D Array(1D array=w921, element="账号:") -> (index of element=w919:i32)  [unwired: 1 in]
        n414 = String Length(string="账号:") -> (length=w915:i32)
        n415 = String Length(string="密码:") -> (length=w914:i32)
        n416 = Equal?(x=w915, y=w913) -> (x = y?=w912:bool)
        n417 = Equal?(x=w914, y=w913) -> (x = y?=w911:bool)
        n418 = Equal?(x=w919, y=-1) -> (x = y?=w908:bool)
        n419 = Index Array(array=w917, index (row)=w919, index (col)=1 ("索引 (列)")) -> (element=w916:string)
        n420 = Equal?(x=w916, y="密码:") -> (x = y?=w907:bool)
        n421 = Or(x=w912, y=w911) -> (x .or. y?=w910:bool)
        n422 = case shown="假" w910 {
          tunnel: [w933 "Idle" ("State(s) at Back (\"\")")] -> w909
          tunnel: w908 -> [w934 _]
          tunnel: w907 -> [w932 _]
          tunnel: w906 -> [w931 w954]
          tunnel: [w930 w954] -> w905
          tunnel: "账号:" -> [w929 _]
          frame False {
            n423 = case shown="假" w934 {
              tunnel: [w938 "Idle"] -> w933
              tunnel: w932 -> [w939 _]
              tunnel: w931 -> [w937 w951]
              tunnel: [w936 w951] -> w930
              tunnel: w929 -> [w935 _]
              frame False {
                n424 = case shown="真" w939 {
                  tunnel: ["Idle" "Idle"] -> w938
                  tunnel: w937 -> [w940 w947]
                  tunnel: [w940 w946] -> w936
                  tunnel: w935 -> [_ w944]
                  frame False {
                    n425 = One Button Dialog(message="用户名或密码错误" ("消息")) -> ()  [unwired: 1 in, 1 out]
                  }
                  frame True {
                    n426 = Bundle By Name(cluster=w947, "用户名"=w944) -> (w946:T15)
                    n427 = One Button Dialog(message="登录成功" ("消息")) -> ()  [unwired: 1 in, 1 out]
                    n428 = local write "选项卡控件"(选项卡枚举."主界面" ("枚举")) -> ()
                    n429 = property on="选项卡控件" class="TabCtl (严格)"("PageSelVis"=TRUE ("选项卡标签显示可见？")) -> ()  [unwired: 2 in, 2 out]
                    n430 = property on="Toolbar 5" class="Clust (严格)"("Visible"=TRUE ("可见")) -> ()  [unwired: 2 in, 2 out]
                    "玩家" <- w944
                  }
                }
              }
              frame True {
                n431 = One Button Dialog(message="用户名不存在" ("消息")) -> ()  [unwired: 1 in, 1 out]
              }
            }
          }
          frame True {
            n432 = One Button Dialog(message="用户名或密码不能为空！" ("消息")) -> ()  [unwired: 1 in, 1 out]
          }
        }
        n433 = call <vilib>:"Add State(s) to Queue__JKI_lib_State_Machine.vi"("State(s) in (\"\")"=w928, "State(s) at Back (\"\")"=w909) -> ("States Out"=w927:string)  [unwired: 13 in]
      }
      frame "User: Exit" {
        # "Your code here.\n(You can make a copy of, or modify, this frame)"
        n434 = call <vilib>:"Add State(s) to Queue__JKI_lib_State_Machine.vi"("State(s) in (\"\")"=w963) -> ("States Out"=w962:string)  [unwired: 14 in]
      }
      frame "---------- Game ----------" {
        # "Template Separator\n(You can make a copy of, or modify, this frame)"
        n435 = call <vilib>:"Add State(s) to Queue__JKI_lib_State_Machine.vi"("State(s) in (\"\")"=w970) -> ("States Out"=w969:string)  [unwired: 14 in]
      }
      frame "Game: Select_Difficulty" {
        # "Template Separator\n(You can make a copy of, or modify, this frame)"
        n436 = Concatenate Strings("欢迎" ("message"), "选择难度" ("string"), "\r") -> (w982:string)
        n437 = call <vilib>:"Three Button Dialog.vi"("Allow user to close window? (TRUE)"=FALSE, "Right Button Text (\"Cancel\")"="困难" ("Right Button Text (\"Cancel\")"), "Center Button Text (\"No\")"="中等" ("Center Button Text (\"No\")"), "Left Button Text (\"Yes\")"="简单" ("Left Button Text (\"Yes\")"), "message"=w982) -> ("Which Button?"=w980:T22)  [unwired: 6 in]
        n438 = case shown="\"Right Button\"" w980 {
          tunnel: [727 303 100] -> w975
          tunnel: [750 350 150] -> w976
          tunnel: ["简单" "中等" "困难"] -> w977
          frame "Left Button", Default {
          }
          frame "Center Button" {
          }
          frame "Right Button" {
          }
        }
        "超时时间" <- w975
        "闪烁间隔" <- w976
        "难度" <- w977
        n439 = Bundle By Name(cluster=w979, "难度_保存"=w977, "闪烁间隔_保存"=w976, "超时时间_保存"=w975) -> (w978:T15)
        n440 = call <vilib>:"Add State(s) to Queue__JKI_lib_State_Machine.vi"("State(s) in (\"\")"=w991, "State(s) at Back (\"\")"="Game: Twinkle" ("State(s) at Back (\"\")")) -> ("States Out"=w990:string)  [unwired: 13 in]
      }
      frame "Game: Twinkle" {
        # "0、1、2、3对应上右下左四个灯"
        # "根据回合选择亮灯顺序"
        # "Template Separator\n(You can make a copy of, or modify, this frame)"
        n441 = Array Subset(array=w1006, index=0 ("索引"), length="亮灯次数") -> (w1004:u64[])
        n442 = for {
          tunnel: w1004 -> [w1012] mode=indexing
          stop <- w1013 stop-if-true
          n443 = case shown="3" w1012 {
            frame 0, Default {
              n444 = stacked-sequence {
                frame #0 {
                  n445 = local write "游戏界面_上"(TRUE ("上")) -> ()
                }
                frame #1 {
                  n446 = local read "闪烁间隔"() -> (w1015:i32)
                  n447 = Wait (ms)(milliseconds to wait=w1015) -> ()  [unwired: 1 out]
                }
                frame #2 {
                  n448 = local write "游戏界面_上"(FALSE ("上")) -> ()
                }
                frame #3 {
                  n449 = Wait (ms)(milliseconds to wait=u32 250 ("等待时间（毫秒）")) -> ()  [unwired: 1 out]
                }
              }
            }
            frame 1 {
              n450 = stacked-sequence {
                frame #0 {
                  n451 = local write "游戏界面_右"(TRUE ("上")) -> ()
                }
                frame #1 {
                  n452 = local read "闪烁间隔"() -> (w1019:i32)
                  n453 = Wait (ms)(milliseconds to wait=w1019) -> ()  [unwired: 1 out]
                }
                frame #2 {
                  n454 = local write "游戏界面_右"(FALSE ("上")) -> ()
                }
                frame #3 {
                  n455 = Wait (ms)(milliseconds to wait=u32 250 ("等待时间（毫秒）")) -> ()  [unwired: 1 out]
                }
              }
            }
            frame 2 {
              n456 = stacked-sequence {
                frame #0 {
                  n457 = local write "游戏界面_下"(TRUE ("上")) -> ()
                }
                frame #1 {
                  n458 = local read "闪烁间隔"() -> (w1023:i32)
                  n459 = Wait (ms)(milliseconds to wait=w1023) -> ()  [unwired: 1 out]
                }
                frame #2 {
                  n460 = local write "游戏界面_下"(FALSE ("上")) -> ()
                }
                frame #3 {
                  n461 = Wait (ms)(milliseconds to wait=u32 250 ("等待时间（毫秒）")) -> ()  [unwired: 1 out]
                }
              }
            }
            frame 3 {
              n462 = stacked-sequence {
                frame #0 {
                  n463 = local write "游戏界面_左"(TRUE ("上")) -> ()
                }
                frame #1 {
                  n464 = local read "闪烁间隔"() -> (w1027:i32)
                  n465 = Wait (ms)(milliseconds to wait=w1027) -> ()  [unwired: 1 out]
                }
                frame #2 {
                  n466 = local write "游戏界面_左"(FALSE ("上")) -> ()
                }
                frame #3 {
                  n467 = Wait (ms)(milliseconds to wait=u32 250 ("等待时间（毫秒）")) -> ()  [unwired: 1 out]
                }
              }
            }
          }
          n468 = local read "游戏界面_结束"() -> (w1013:bool)
        }
        n469 = call <vilib>:"Add State(s) to Queue__JKI_lib_State_Machine.vi"("State(s) in (\"\")"=w1011, "State(s) at Back (\"\")"="Game: start counting" ("State(s) at Back (\"\")")) -> ("States Out"=w1010:string)  [unwired: 13 in]
      }
      frame "Game: start counting" {
        # "Template Separator\n(You can make a copy of, or modify, this frame)"
        n470 = local write "是否开始计时？"(TRUE ("是否开始计时？")) -> ()
        n471 = local write "键盘启用"(TRUE ("键盘启用")) -> ()
        n472 = Wait (ms)(milliseconds to wait=u32 50 ("等待时间（毫秒）")) -> ()  [unwired: 1 out]
        n473 = call <vilib>:"Add State(s) to Queue__JKI_lib_State_Machine.vi"("State(s) in (\"\")"=w1040, "State(s) at Back (\"\")"="Idle" ("State(s) at Back (\"\")")) -> ("States Out"=w1039:string)  [unwired: 13 in]
      }
      frame "Game: Option" {
        # "提取要判断的灯号"
        # "判断是否超时"
        # "判断点亮的灯是否正确\n+1使判断的索引每循环一次向后移一位"
        # "判断是否按完"
        # "Template Separator\n(You can make a copy of, or modify, this frame)"
        n474 = Decrement(x=w1042) -> (x-1=w1052:i32)
        n475 = Index Array(array=w1051, index=w1052) -> (element=w1050:u64)
        n476 = case shown="\"黄\"" w1041 {
          tunnel: w1050 -> [_ _ _ _ w1083 w1091 w1099 w1109]
          tunnel: w1042 -> [w1069 w1074 w1077 _ w1080 w1088 w1096 w1104]
          tunnel: [w1069 w1074 w1077 w1079 w1082 w1090 w1098 w1106] -> w1047
          tunnel: [0 0 0 w1079 w1080 w1088 w1096 w1104] -> w1048
          tunnel: ["Game: Read" "Game: Save" "Idle" "Game: Exit" w1081 w1089 w1097 w1105] -> w1046
          frame "读档" {
          }
          frame "存档" {
          }
          frame "按错", Default {
          }
          frame "退出" {
            w1079 = 0
          }
          frame "黄" {
            n477 = Equal?(x=w1083, y=u64 3) -> (x = y?=w1085:bool)
            n478 = Increment(x=w1080) -> (x+1=w1082:i32)
            n479 = case shown="假" w1085 {
              tunnel: ["Game: Exit" "Idle"] -> w1081
              frame False {
              }
              frame True {
              }
            }
          }
          frame "红" {
            n480 = Equal?(x=w1091, y=u64 2) -> (x = y?=w1093:bool)
            n481 = Increment(x=w1088) -> (x+1=w1090:i32)
            n482 = case shown="真" w1093 {
              tunnel: ["Game: Exit" "Idle"] -> w1089
              frame False {
              }
              frame True {
              }
            }
          }
          frame "蓝" {
            n483 = Equal?(x=w1099, y=u64 1) -> (x = y?=w1101:bool)
            n484 = Increment(x=w1096) -> (x+1=w1098:i32)
            n485 = case shown="真" w1101 {
              tunnel: ["Game: Exit" "Idle"] -> w1097
              frame False {
              }
              frame True {
              }
            }
          }
          frame "绿" {
            n486 = Equal?(x=w1109, y=u64 0) -> (x = y?=w1108:bool)
            n487 = Increment(x=w1104) -> (x+1=w1106:i32)
            n488 = case shown="真" w1108 {
              tunnel: ["Game: Exit" "Idle"] -> w1105
              frame False {
              }
              frame True {
              }
            }
          }
        }
        n489 = local read "亮灯次数"() -> (w1049:i32)
        n490 = Greater Or Equal?(x=w1048, y=w1049) -> (x >= y?=w1043:bool)
        n491 = local read "游戏界面_时间到"() -> (w1045:bool)
        n492 = case shown="真" w1045 {
          tunnel: w1046 -> [w1059 _]
          tunnel: w1043 -> [w1058 _]
          tunnel: [w1057 "Game: Exit"] -> w1044
          frame False {
            n493 = case shown="\"Game: Option\", 默认" w1059 {
              selector: w1059 -> [w1061 w1065 w1066 w1067]
              tunnel: w1058 -> [w1062 _ _ _]
              tunnel: [w1060 w1065 w1066 w1067] -> w1057
              frame "Game: Option", Default {
                n494 = case shown="真" w1062 {
                  tunnel: [w1063 "Game: stop counting"] -> w1060
                  tunnel: w1061 -> [w1063 _]
                  frame False {
                  }
                  frame True {
                    # "下一回合"
                  }
                }
              }
              frame "Game: Read" {
              }
              frame "Game: Save" {
              }
              frame "Game: Exit" {
              }
            }
          }
          frame True {
          }
        }
        n495 = call <vilib>:"Add State(s) to Queue__JKI_lib_State_Machine.vi"("State(s) in (\"\")"=w1056, "State(s) at Back (\"\")"=w1044) -> ("States Out"=w1055:string)  [unwired: 13 in]
      }
      frame "Game: Exit" {
        # "Template Separator\n(You can make a copy of, or modify, this frame)"
        n496 = local read "分数"() -> (w1127:i32)
        n497 = local read "难度"() -> (w1123:string)
        n498 = Number To Decimal String(number=w1127) -> (decimal integer string=w1120:string)  [unwired: 1 in]
        n499 = Concatenate Strings("游戏结束！", "\n", "难度：" ("字符串"), w1123, "\n", "得分：" ("字符串"), w1120) -> (w1117:string)
        n500 = Two Button Dialog(message=w1117, 1:"结束" ("F按钮名称（“取消”）"), 2:"重新开始" ("T按钮名称（“确定”）")) -> (T button?=w1114:bool)
        n501 = case shown="假" w1114 {
          tunnel: ["Game: TOP10" ("State(s) at Back (\"\")") "UI: Initialize\nGame: Select_Difficulty" ("State(s) at Back (\"\")")] -> w1113
          frame False {
            n502 = property on="TOP10_退出" class="Bool (严格)"("Visible"=TRUE ("可见")) -> ()  [unwired: 2 in, 2 out]
            n503 = property on="TOP10_返回" class="Bool (严格)"("Visible"=TRUE ("可见")) -> ()  [unwired: 2 in, 2 out]
            n504 = local write "选项卡控件"(选项卡枚举."TOP10" ("枚举")) -> ()
          }
          frame True {
          }
        }
        n505 = call <vilib>:"Add State(s) to Queue__JKI_lib_State_Machine.vi"("State(s) in (\"\")"=w1131, "State(s) at Back (\"\")"=w1113) -> ("States Out"=w1130:string)  [unwired: 13 in]
      }
      frame "Game: stop counting" {
        # "Template Separator\n(You can make a copy of, or modify, this frame)"
        n506 = local read "分数"() -> (w1144:i32)
        n507 = Increment(x=w1144) -> (x+1=w1137:i32)
        n508 = local write "分数"(w1137) -> ()
        n509 = local read "亮灯次数"() -> (w1143:i32)
        n510 = Increment(x=w1143) -> (x+1=w1147:i32)
        n511 = local write "亮灯次数"(w1147) -> ()
        n512 = local write "是否开始计时？"(FALSE ("是否开始计时？")) -> ()
        n513 = Bundle By Name(cluster=w1145, "积分_保存"=w1144, "亮灯次数_保存"=w1143, "积分_排名"=w1137) -> (w1142:T15)
        n514 = Number To Decimal String(number=w1137) -> (decimal integer string=w1149:string)  [unwired: 1 in]
        n515 = local read "难度"() -> (w1151:string)
        n516 = Concatenate Strings(w1151, "模式：" ("字符串"), w1149, "分" ("字符串")) -> (→"难度：分数":string)
        n517 = Wait (ms)(milliseconds to wait=u32 150 ("等待时间（毫秒）")) -> ()  [unwired: 1 out]
        n518 = call <vilib>:"Add State(s) to Queue__JKI_lib_State_Machine.vi"("State(s) in (\"\")"=w1156, "State(s) at Back (\"\")"="Game: Twinkle" ("State(s) at Back (\"\")")) -> ("States Out"=w1155:string)  [unwired: 13 in]
      }
      frame "Game: Save" {
        # "Template Separator\n(You can make a copy of, or modify, this frame)"
        n519 = flat-sequence {
          tunnel: w1163 -> [w1176]
          tunnel: [w1169] -> w1159
          tunnel: w1158 -> [w1168]
          tunnel: [w1167] -> w1157
          tunnel: w1159 -> [_]
          tunnel: w1157 -> [w1180]
          frame #0 {
            n520 = Unbundle By Name(w1176) -> ("难度_保存"=w1175:string, "亮灯次数_保存"=w1173:i32, "超时时间_保存"=w1172:i32, "闪烁间隔_保存"=w1171:i32, "积分_保存"=w1170:i32)
            n521 = case shown="\"简单\"" w1175 {
              tunnel: [2 0 1] -> w1174
              frame "困难", Default {
              }
              frame "简单" {
              }
              frame "中等" {
              }
            }
            n522 = Build Array(w1174, w1173, w1172, w1171, w1170) -> (w1169:i32[])
            n523 = Build Array(w1168, w1169) -> (w1167:u64[][])
          }
          frame #1 {
            n524 = call "文件对话框"("default name"="请选择保存的位置") -> ("selected path"=w1182:path)  [unwired: 11 in, 3 out]
            n525 = call-poly <vilib>:"Write Delimited Spreadsheet.vi"("file path (dialog if empty)"=w1182, "2D data"=w1180) -> ()  [unwired: 12 in, 2 out]
          }
          frame #2 {
            n526 = One Button Dialog(message="保存成功" ("消息")) -> ()  [unwired: 1 in, 1 out]
            n527 = local write "选项卡控件"(选项卡枚举."主界面" ("枚举")) -> ()
          }
        }
        n528 = local write "是否开始计时？"(FALSE ("是否开始计时？")) -> ()
        n529 = call <vilib>:"Add State(s) to Queue__JKI_lib_State_Machine.vi"("State(s) in (\"\")"=w1166) -> ("States Out"=w1165:string)  [unwired: 14 in]
      }
      frame "Game: Read" {
        w1193 = 1 ("禁用的索引 (行)")
        # "第一行第二列数据"
        # "第一行第一列数据"
        # "第0行数据为保存的目标数组"
        # "Template Separator\n(You can make a copy of, or modify, this frame)"
        n530 = call "文件对话框2"("default name"="请选择要读取的存档") -> ("selected path"=w1202:path)  [unwired: 11 in, 3 out]
        n531 = call-poly <vilib>:"Read Delimited Spreadsheet.vi"("file path (dialog if empty)"=w1202) -> ("all rows"=w1190:i64[][], "first row"=w1201:i64[])  [unwired: 9 in, 4 out]
        n532 = Index Array(array=w1190, index (row)=w1193, index (col)=0 ("禁用的索引 (列)")) -> (element=w1192:i64)
        n533 = Index Array(array=w1190, index (row)=w1193, index (col)=1 ("禁用的索引 (列)")) -> (element=w1189:i64)
        n534 = Index Array(array=w1190, index (row)=w1193, index (col)=2 ("禁用的索引 (列)")) -> (element=w1188:i64)
        n535 = Index Array(array=w1190, index (row)=w1193, index (col)=3 ("禁用的索引 (列)")) -> (element=w1187:i64)
        n536 = Index Array(array=w1190, index (row)=w1193, index (col)=4 ("禁用的索引 (列)")) -> (element=w1186:i64)
        n537 = local write "闪烁间隔"(w1187) -> ()
        n538 = local write "超时时间"(w1188) -> ()
        n539 = local write "亮灯次数"(w1189) -> ()
        n540 = case shown="2" w1192 {
          tunnel: ["简单" "中等" "困难"] -> w1191
          frame 0, Default {
          }
          frame 1 {
          }
          frame 2 {
          }
        }
        n541 = local write "分数"(w1186) -> ()
        n542 = local write "难度"(w1191) -> ()
        n543 = local write "选项卡控件"(选项卡枚举."游戏界面" ("枚举")) -> ()
        n544 = To Unsigned Quad Integer(1:w1201) -> (0:w1200:u64[])
        n545 = call <vilib>:"Add State(s) to Queue__JKI_lib_State_Machine.vi"("State(s) in (\"\")"=w1209, "State(s) at Back (\"\")"="Game: Twinkle" ("State(s) at Back (\"\")")) -> ("States Out"=w1208:string)  [unwired: 13 in]
      }
      frame "Game: TOP10" {
        # "Template Separator\n(You can make a copy of, or modify, this frame)"
        n546 = call <vilib>:"Application Directory.vi"() -> ("Application Directory"=w1214:path)
        n547 = flat-sequence {
          tunnel: w1215 -> [w1231]
          tunnel: w1214 -> [w1222]
          tunnel: w1214 -> [w1288]
          frame #0 {
            # "判断是否为新用户"
            # "将用户名与积分创建为一个数组"
            n548 = Unbundle By Name(w1231) -> ("难度_保存"=w1230:string, "用户名"=w1229:string, "积分_排名"=w1228:i32)
            n549 = case shown="\"中等\"" w1230 {
              tunnel: w1229 -> [w1245 w1258 w1271]
              tunnel: w1228 -> [w1246 w1260 w1272]
              tunnel: w1222 -> [w1247 w1261 w1273]
              tunnel: [w1242 w1257 w1268] -> w1227
              tunnel: [w1240 w1256 w1266] -> w1223
              tunnel: [w1241 w1255 w1267] -> w1226
              tunnel: [w1244 w1254 w1270] -> w1225
              tunnel: [w1243 w1253 w1269] -> w1224
              frame "简单", Default {
                n550 = Number To Decimal String(number=w1246) -> (decimal integer string=w1248:string)  [unwired: 1 in]
                n551 = Build Array(w1245, w1248) -> (w1243:string[])
                n552 = Build Path(base path=w1247, name or relative path="排名简单.txt" ("名称或相对路径")) -> (appended path=w1240:path)
                n553 = call-poly <vilib>:"Read Delimited Spreadsheet.vi"("file path (dialog if empty)"=w1240) -> ("all rows"=w1241:string[][])  [unwired: 9 in, 5 out]
                n554 = Index Array(array=w1241, index (col)=0 ("禁用的索引 (列)")) -> (element=w1250:string[])  [unwired: 1 in]
                n555 = Search 1D Array(1D array=w1250, element=w1245) -> (index of element=w1244:i32)  [unwired: 1 in]
                n556 = Equal?(x=w1244, y=-1) -> (x = y?=w1242:bool)
              }
              frame "中等" {
                n557 = Number To Decimal String(number=w1260) -> (decimal integer string=w1259:string)  [unwired: 1 in]
                n558 = Build Array(w1258, w1259) -> (w1253:string[])
                n559 = Build Path(base path=w1261, name or relative path="排名中等.txt" ("名称或相对路径")) -> (appended path=w1256:path)
                n560 = call-poly <vilib>:"Read Delimited Spreadsheet.vi"("file path (dialog if empty)"=w1256) -> ("all rows"=w1255:string[][])  [unwired: 9 in, 5 out]
                n561 = Index Array(array=w1255, index (col)=0 ("禁用的索引 (列)")) -> (element=w1263:string[])  [unwired: 1 in]
                n562 = Search 1D Array(1D array=w1263, element=w1258) -> (index of element=w1254:i32)  [unwired: 1 in]
                n563 = Equal?(x=w1254, y=-1) -> (x = y?=w1257:bool)
              }
              frame "困难" {
                n564 = Number To Decimal String(number=w1272) -> (decimal integer string=w1274:string)  [unwired: 1 in]
                n565 = Build Array(w1271, w1274) -> (w1269:string[])
                n566 = Build Path(base path=w1273, name or relative path="排名困难.txt" ("名称或相对路径")) -> (appended path=w1266:path)
                n567 = call-poly <vilib>:"Read Delimited Spreadsheet.vi"("file path (dialog if empty)"=w1266) -> ("all rows"=w1267:string[][])  [unwired: 9 in, 5 out]
                n568 = Index Array(array=w1267, index (col)=0 ("禁用的索引 (列)")) -> (element=w1276:string[])  [unwired: 1 in]
                n569 = Search 1D Array(1D array=w1276, element=w1271) -> (index of element=w1270:i32)  [unwired: 1 in]
                n570 = Equal?(x=w1270, y=-1) -> (x = y?=w1268:bool)
              }
            }
            n571 = case shown="假" w1227 {
              tunnel: w1223 -> [w1234 w1239]
              tunnel: w1226 -> [w1236 _]
              tunnel: w1225 -> [w1233 _]
              tunnel: w1224 -> [w1235 w1238]
              frame False {
                n572 = Replace Array Subset(array=w1236, new element=w1235, index (row)=w1233) -> (w1232:string[][])  [unwired: 1 in]
                n573 = call-poly <vilib>:"Write Delimited Spreadsheet.vi"("file path (dialog if empty)"=w1234, "2D data"=w1232) -> ()  [unwired: 12 in, 2 out]
              }
              frame True {
                n574 = call-poly <vilib>:"Write Delimited Spreadsheet.vi"("file path (dialog if empty)"=w1239, "1D data"=w1238, "append to file? (new file:F)"=TRUE) -> ()  [unwired: 11 in, 2 out]
              }
            }
          }
          frame #1 {
            n575 = Build Path(base path=w1288, name or relative path="排名简单.txt" ("名称或相对路径")) -> (appended path=w1287:path)
            n576 = Build Path(base path=w1288, name or relative path="排名中等.txt" ("名称或相对路径")) -> (appended path=w1286:path)
            n577 = Build Path(base path=w1288, name or relative path="排名困难.txt" ("名称或相对路径")) -> (appended path=w1285:path)
            n578 = call-poly <vilib>:"Read Delimited Spreadsheet.vi"("file path (dialog if empty)"=w1287) -> ("all rows"=w1284:string[][])  [unwired: 9 in, 5 out]
            n579 = call-poly <vilib>:"Read Delimited Spreadsheet.vi"("file path (dialog if empty)"=w1286) -> ("all rows"=w1283:string[][])  [unwired: 9 in, 5 out]
            n580 = call-poly <vilib>:"Read Delimited Spreadsheet.vi"("file path (dialog if empty)"=w1285) -> ("all rows"=w1282:string[][])  [unwired: 9 in, 5 out]
            n581 = call "排序.vi"("排序前"=w1284) -> ("排序后"=→"玩家                      积分          简单":string[][])
            n582 = call "排序.vi"("排序前"=w1283) -> ("排序后"=→"玩家                      积分          中等":string[][])
            n583 = call "排序.vi"("排序前"=w1282) -> ("排序后"=→"玩家                      积分          困难":string[][])
          }
        }
        n584 = property on="AniGIF" class="AXCont"("Visible"=FALSE ("可见")) -> ()  [unwired: 2 in, 2 out]
        n585 = call <vilib>:"Add State(s) to Queue__JKI_lib_State_Machine.vi"("State(s) in (\"\")"=w1221) -> ("States Out"=w1220:string)  [unwired: 14 in]
      }
    }
  }
  n586 = disable-structure shown="禁用" {
    frame Disabled {
      n587 = while "While循环" {
        shift-right: [w1298] -> _
        shift-left: enum16{"倒计时", "初始化"}."初始化" -> [w1299]
        stop <- w1293 stop-if-true
        # "倒计时"
        n588 = local read "亮灯次数"() -> (w1295:i32)
        n589 = Increment(x=w1295) -> (x+1=w1294:i32)
        n590 = local read "超时时间"() -> (w1297:i32)
        n591 = Multiply(x=w1297, y=w1294) -> (x*y=w1296:i32)
        n592 = case shown="\"倒计时\"" w1299 {
          tunnel: [enum16{"倒计时", "初始化"}."倒计时" enum16{"倒计时", "初始化"}."倒计时"] -> w1298
          tunnel: w1296 -> [w1301 _]
          tunnel: [w1302 FALSE] -> w1293
          frame "倒计时" {
            n593 = case shown="真" "是否开始计时？" {
              tunnel: w1301 -> [_ w1308]
              tunnel: [w1305 w1307] -> w1302
              frame False {
                n594 = local read "游戏界面_结束"() -> (w1304:bool)
                n595 = Or(x=w1304, y=FALSE) -> (x .or. y?=w1305:bool)
              }
              frame True {
                n596 = for {
                  N: w1308 -> [w1317]
                  tunnel: [w1310] -> w1307
                  i -> [w1318]
                  stop <- w1309 stop-if-true
                  n597 = local read "游戏界面_时间到"() -> (w1314:bool)
                  n598 = Subtract(x=w1317, y=w1318) -> (x-y=w1311:i32)
                  "倒计时" <- w1311
                  "x-y" <- w1311
                  n599 = local read "是否开始计时？"() -> (w1315:bool)
                  n600 = Less Or Equal?(x=w1311, y=1) -> (x <= y?=w1312:bool)
                  n601 = Not(x=w1315) -> (.not. x?=w1313:bool)
                  n602 = case shown="真" w1312 {
                    tunnel: w1314 -> [_ w1320]
                    frame False {
                    }
                    frame True {
                      n603 = case shown="真" w1320 {
                        frame False {
                          n604 = property on="游戏界面_时间到" class="Bool (严格)"("Val(Sgnl)"=TRUE ("值(信号)")) -> ()  [unwired: 2 in, 2 out]
                        }
                        frame True {
                          n605 = property on="游戏界面_时间到" class="Bool (严格)"("Val(Sgnl)"=FALSE ("值(信号)")) -> ()  [unwired: 2 in, 2 out]
                        }
                      }
                    }
                  }
                  n606 = Or(x=w1313, y=w1312) -> (x .or. y?=w1309:bool)
                  n607 = local read "游戏界面_结束"() -> (w1310:bool)
                  n608 = Wait (ms)(milliseconds to wait=u32 1 ("等待时间（毫秒）")) -> ()  [unwired: 1 out]
                }
                n609 = property on="倒计时" class="Slide (严格)"("Scale.Maximum"=w1308) -> ()  [unwired: 2 in, 2 out]
              }
            }
          }
          frame "初始化", Default {
            n610 = local write "倒计时"(1111111111 ("滑动杆")) -> ()
          }
        }
      }
    }
    frame Enabled {
    }
  }
